vi "Pick&Place_ladder_shih_v7_center.vi"() -> ()   [LabVIEW 2016]
uses:
  WTF is this.ctl
  Classes/Controllers/I-O/Copy of NI-DAQ Folder/NI-DAQ.lvclass
  D:/INTT/V1/Classes/Controllers/I-O/Copy of I-O Folder/I-O.lvclass
  Classes/Controllers/Dispenser/Copy of Ultimus V2 Folder/Ultimus V2.lvclass
  <vilib>/Analysis/coordinate.llb/2D Cartesian Coordinate Rotation (Scalar).vi
  <vilib>/Utility/file.llb/Read Delimited Spreadsheet (DBL).vi
  <vilib>/Utility/file.llb/Write Delimited Spreadsheet (DBL).vi
  Classes/Controllers/Motion/Copy of Motion Folder/Motion.lvclass
  Classes/Controllers/Camera/Copy of Controller Folder/Controller.lvclass
  <vilib>/Analysis/NI_AALPro.lvlib
  Classes/Controllers/I-O/Copy of I-O Folder/I-O.lvclass
panel:
  in  "pick &place module":i32=1
  in  "txt switch":bool
  in  "offset":dbl[][](array[numeric])=[[0.0, 0.0, 0.0, 0.0], [0.0, 0.0, 0.0, 0.0]]
  out "HPoS_CT":dbl[][](array[numeric]) format="%#_8g"
  out "chip distance by OGP":dbl format="%#_8g"
  out "displacement":dbl[](array[numeric])
  out "gantry position test":dbl[](array[numeric])
  out "stave target position":dbl[](array[numeric])
  out "chip distance by gantry":dbl format="%#_8g"
  out "after SL":dbl[](array[numeric]) format="%#_8g"
  out "after SR":dbl[](array[numeric]) format="%#_8g"
  out "after NL":dbl[](array[numeric]) format="%#_8g"
  out "S chip":dbl[](array[numeric]) format="%#_8g"
  out "N chip":dbl[](array[numeric]) format="%#_8g"
  in  "file path (dialog if empty) 2":path=path "C:/Users/PAGANIS/Desktop/shih cheng wei/OGP/test1-2.txt"
  out "bless from OGP !!! Center of  stave":dbl[](array[numeric])
  out "bless from OGP !! measured stave size":dbl[](array[numeric])
  in  "Bless from OGP":bool
  out "FROM Detail !!! Center of module on stave":dbl[](array[numeric])
  out "FROM Detail !! measured stave size":dbl[](array[numeric])
  in  "Align Stave in detail":bool
  in  "check height?":bool
  in  "Uttimus presssure":i64=10
  out "Status":bool
  out "measured HDI top-left position":dbl[][](array[numeric])
  in  "HDI vacuum channel":i32=18
  in  "vacuum":bool=TRUE
  in  "HDI vacuum":bool
  out "measured stave size":dbl[](array[numeric])
  out "Stave mark":dbl[][](array[numeric])
  out "Center of module on stave":dbl[](array[numeric])
  out "Center of HDI from alignment mark":dbl[](array[numeric])
  out "Measured HDI size":dbl[][](array[numeric])
  out "module positions on stave":T1[][](array[typedef])
  in  "Default Stave dimension":dbl[](array[numeric])=[34.0, 472.0, -0.335295, -0.000320234]
  in  "Default Stave upper left mark":dbl[](array[numeric])=[584.376, 675.576, 70.9882, 0.000840064]
  out "Needle parking position":dbl[](array[numeric])
  in  "Uppler / Lower Stave":bool=TRUE
  out "Gantry current position":dbl[](array[numeric])
  in  "READ Position":bool
  in  "Needle Height Compenstation\n(glue gap)":dbl=0.33
  in  "Needle Alignment":bool
  in  "Parking position":dbl[](array[numeric])=[625.0, 625.0, 0.0, 0.01]
  in  "GOTO":bool
  in  "Default Pickup Tool Position":dbl[][](array[numeric])=[[152.226, 682.729, 36.8129, -0.0151898], [700.0, 800.0, 20.0, 0.01]]
  in  "deposit glue module":i32=1
  in  "Default HDI alignment \nmark position":dbl[](array[numeric])=[448.322, 976.582, 74.9872, 0.000191129]
  in  "Default HDI size":dbl[](array[numeric])=[24.2437, 231.446, -0.099339, 0.000191129]
  out "# of tasks excuted":i32
  out "HDI center positions":dbl[][](array[numeric])
  out "PickupTool \nCenterPosition":dbl[](array[numeric])
  in  "Inititalize":bool
  in  "Pick and place":bool
  in  "Deposit Glue":bool
  in  "Measure Pickup Tools":bool
  in  "Align Stave":bool
  out "default module position on stave":dbl[][](array[numeric])
  in  "Stop":bool
  in  "Measure HDI":bool
  # "Ladder Assembly"
  # "Lower\nmodule"
  # "Upper\nmodule"
  # "+"
  # "="
  # "Sensor 0.32 -> 200 micron glue thickness\nChips 0.37-> 140 micron glue thickness"
  # "ACTIONS"
  # "Stave infomation"
  # "also to switch Upper/Lower"
  # "theta had *-1"
  # "Module infomation"
  # "Pick and Place"
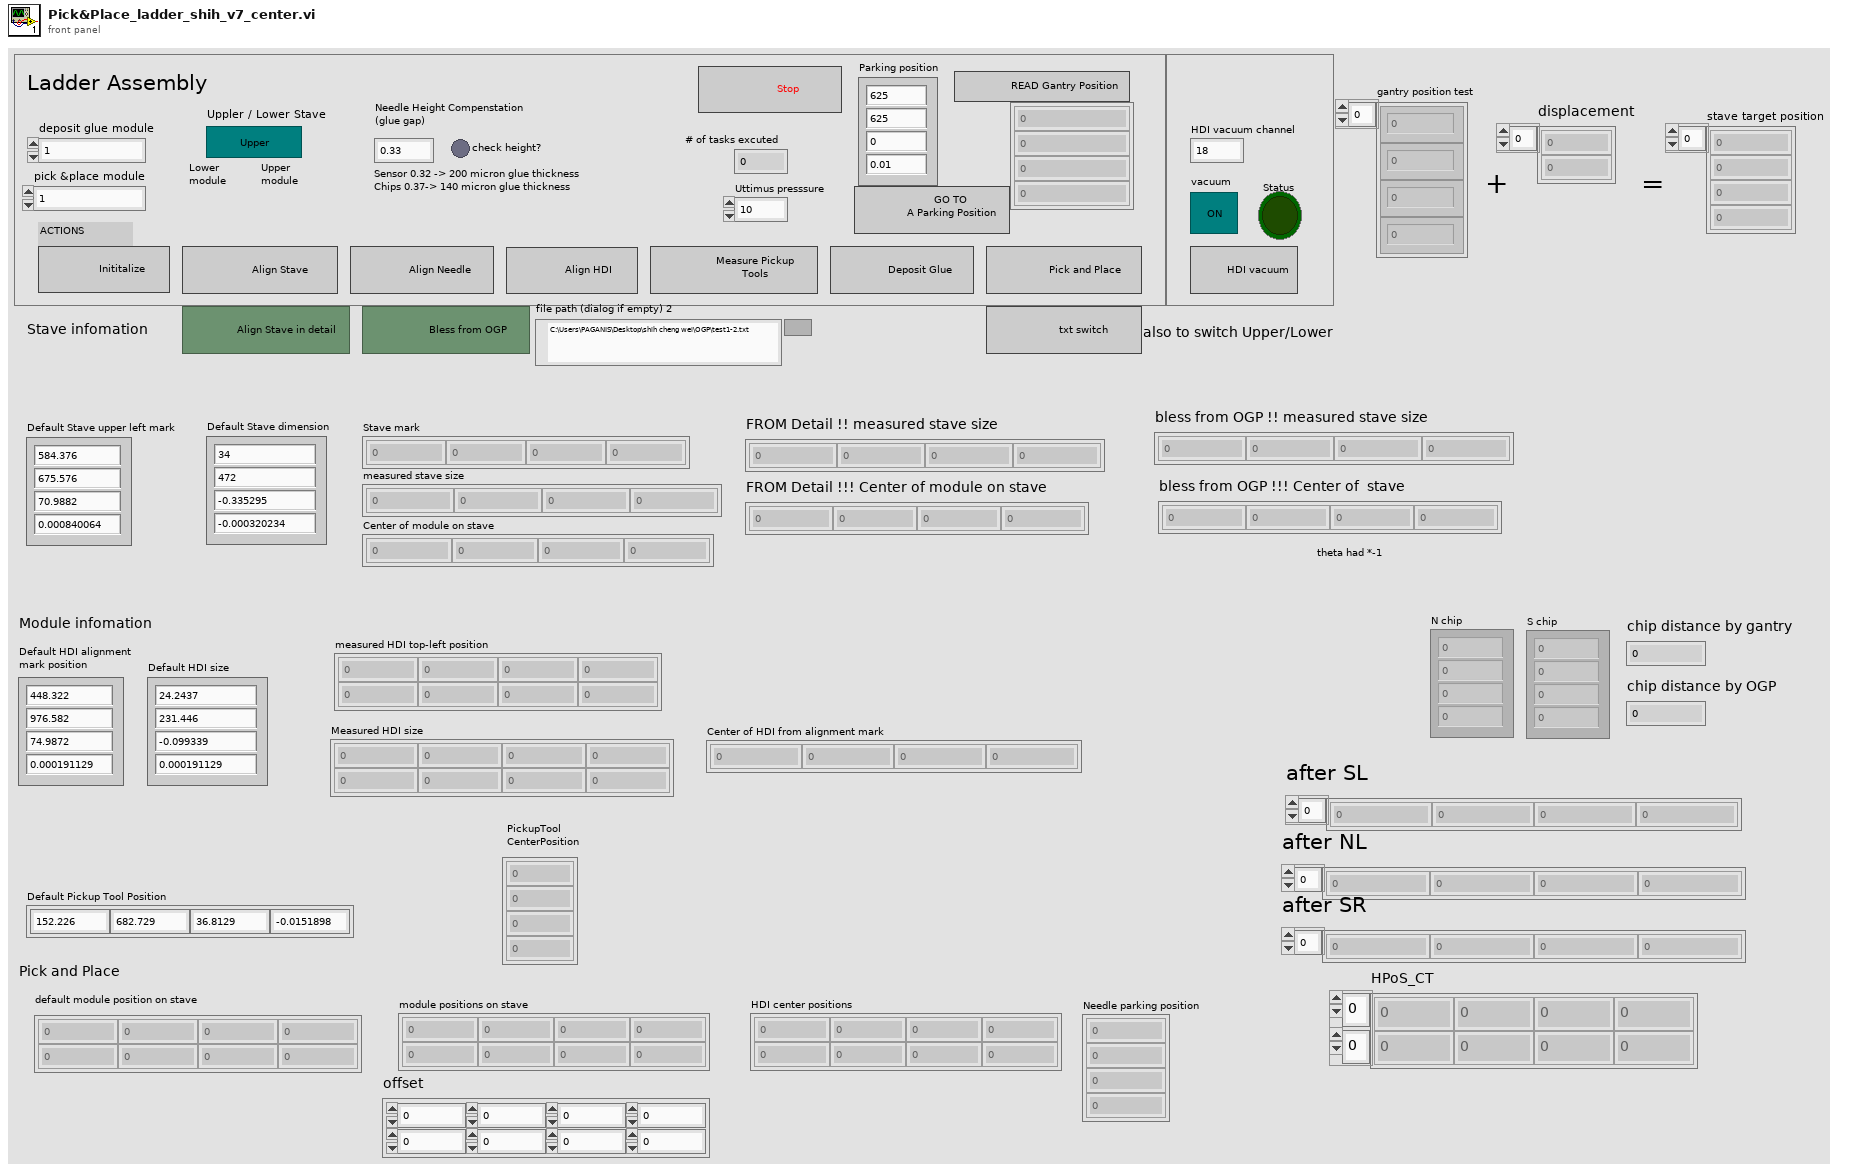
[diagram p1: front panel]
types:
  T1 = typedef "WTF is this.ctl" = dbl
  T2 = typedef "Controller.lvclass/Controllers.ctl" = cluster{"Copy of Motion.lvclass":refnum<class "Motion.lvclass">, "Copy of I-O.lvclass":refnum<class "I-O.lvclass">, "Copy of Dispenser.lvclass":refnum<class "Dispenser.lvclass">}
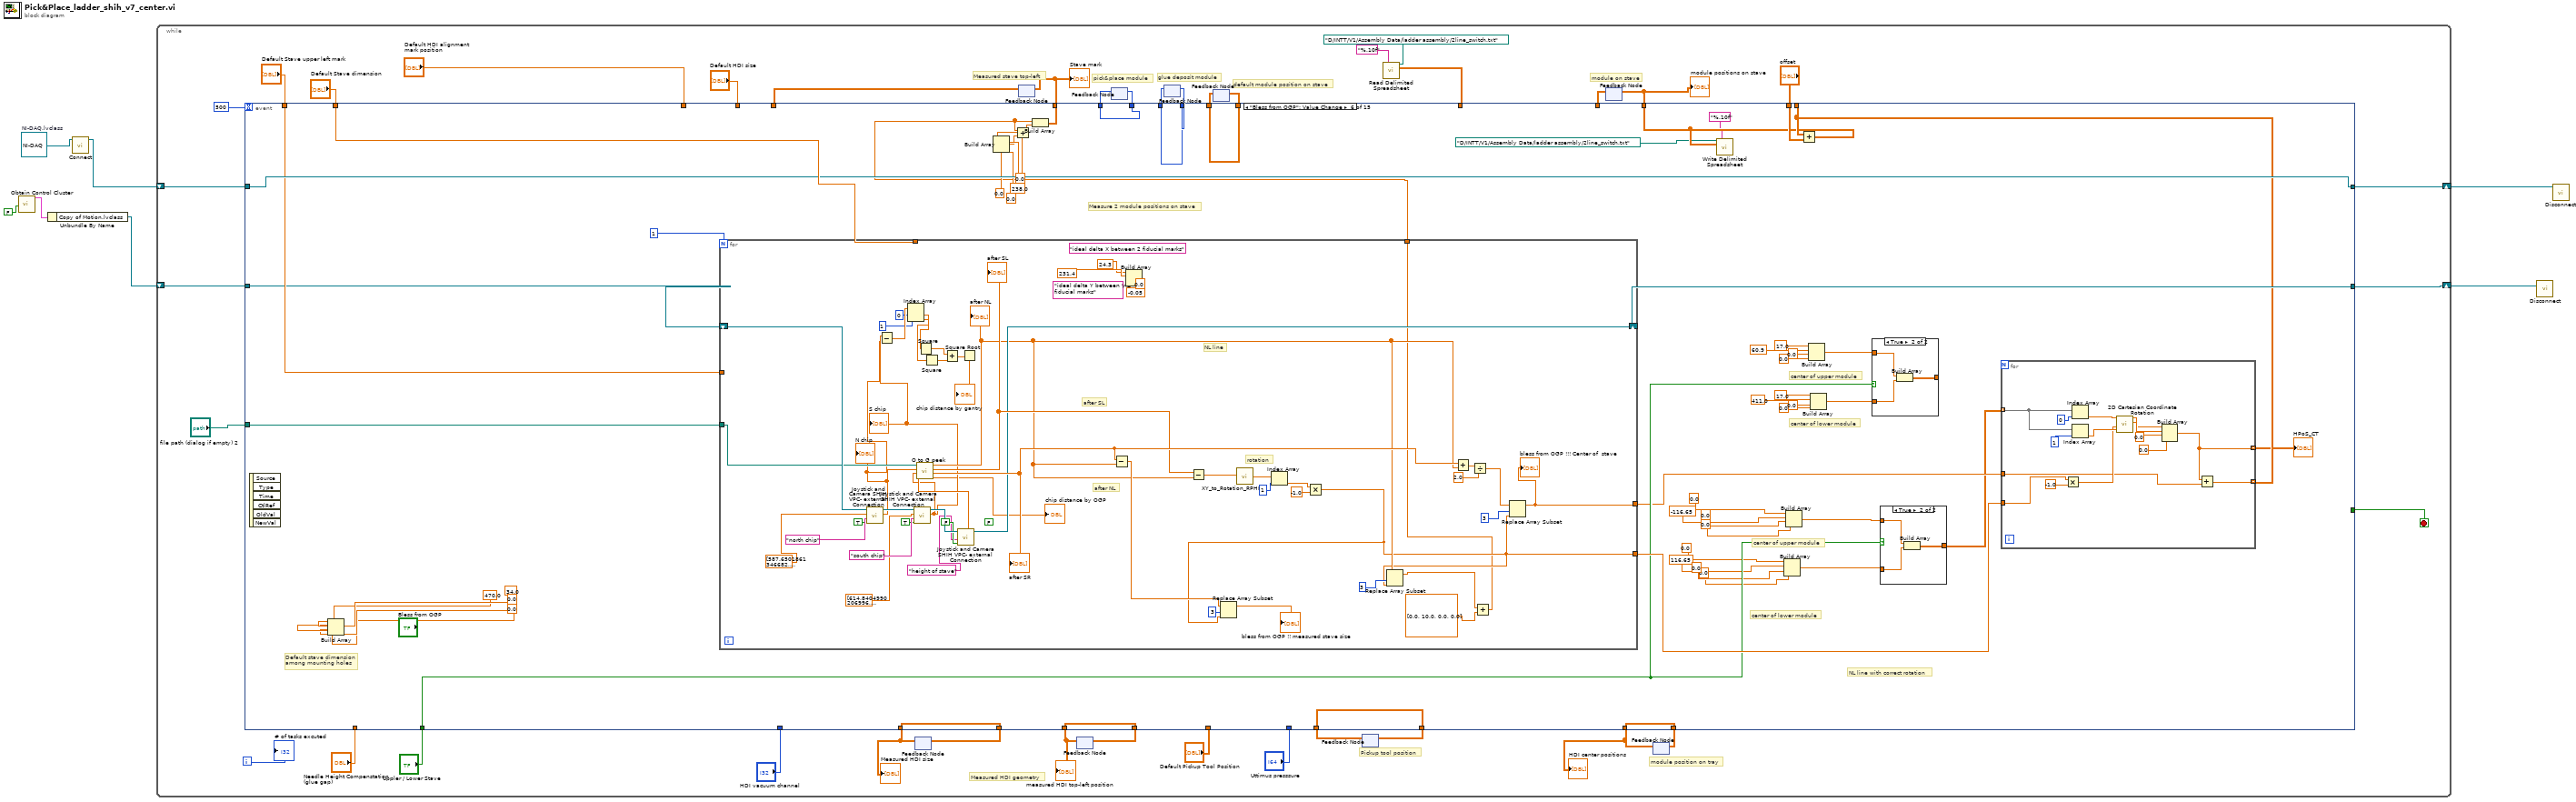
[diagram p0: block diagram]
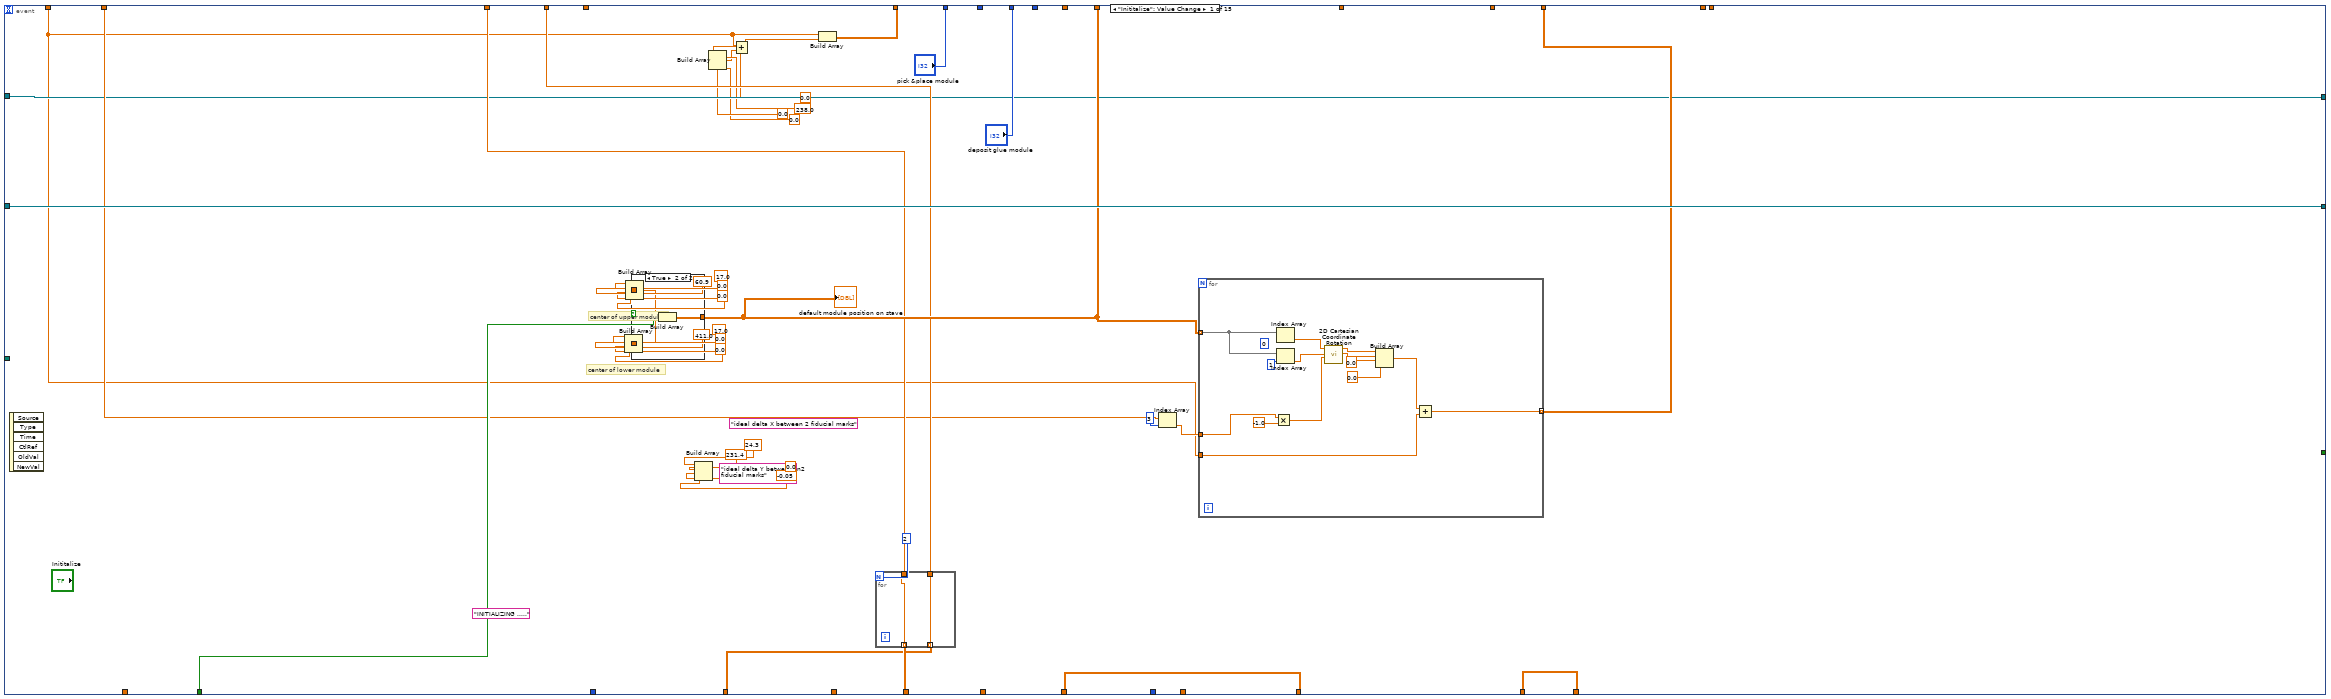
[diagram p2: hidden frame]
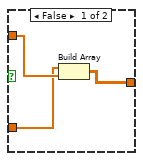
[diagram p3: hidden frame]
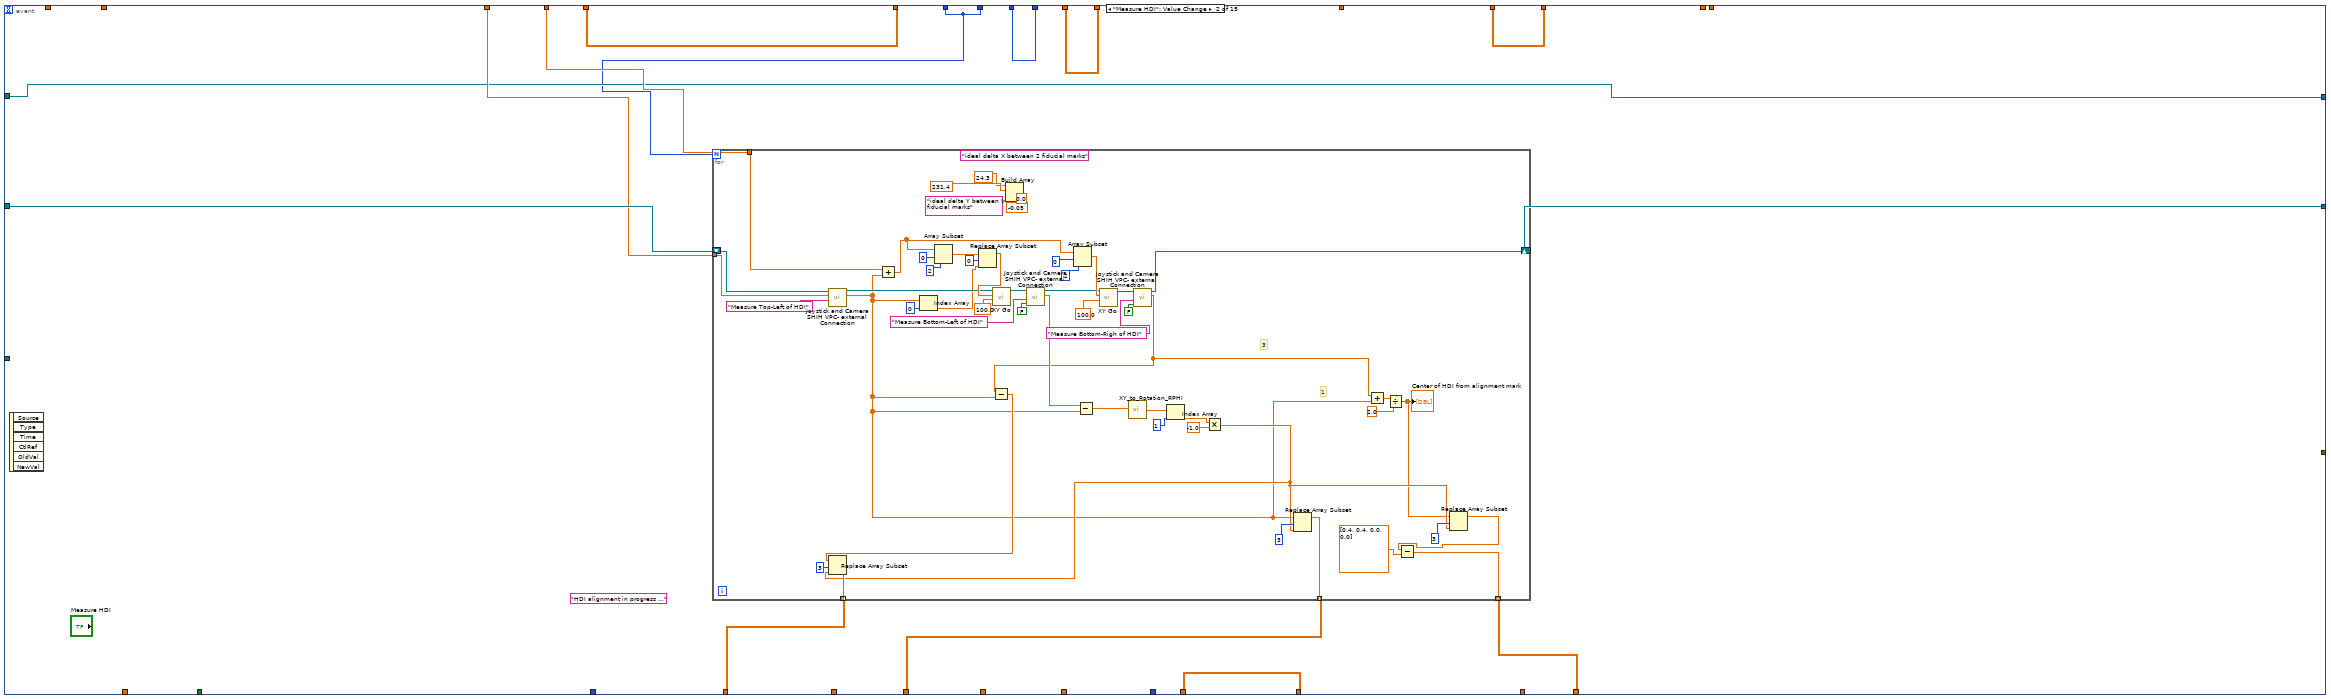
[diagram p4: hidden frame]
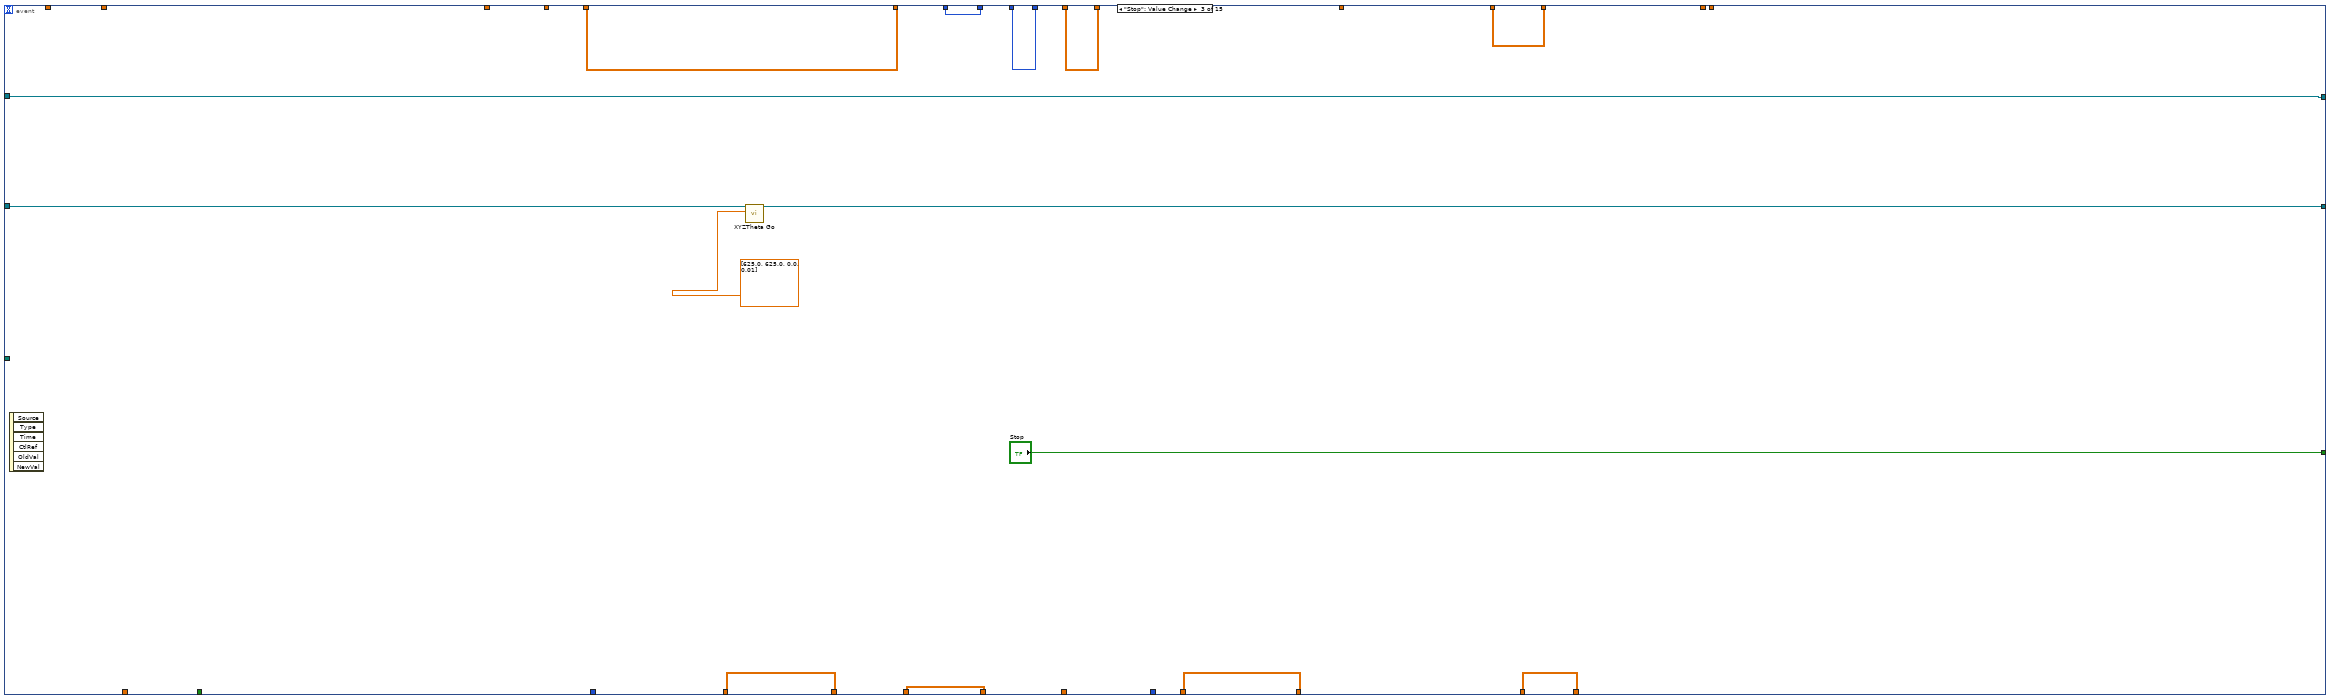
[diagram p5: hidden frame]
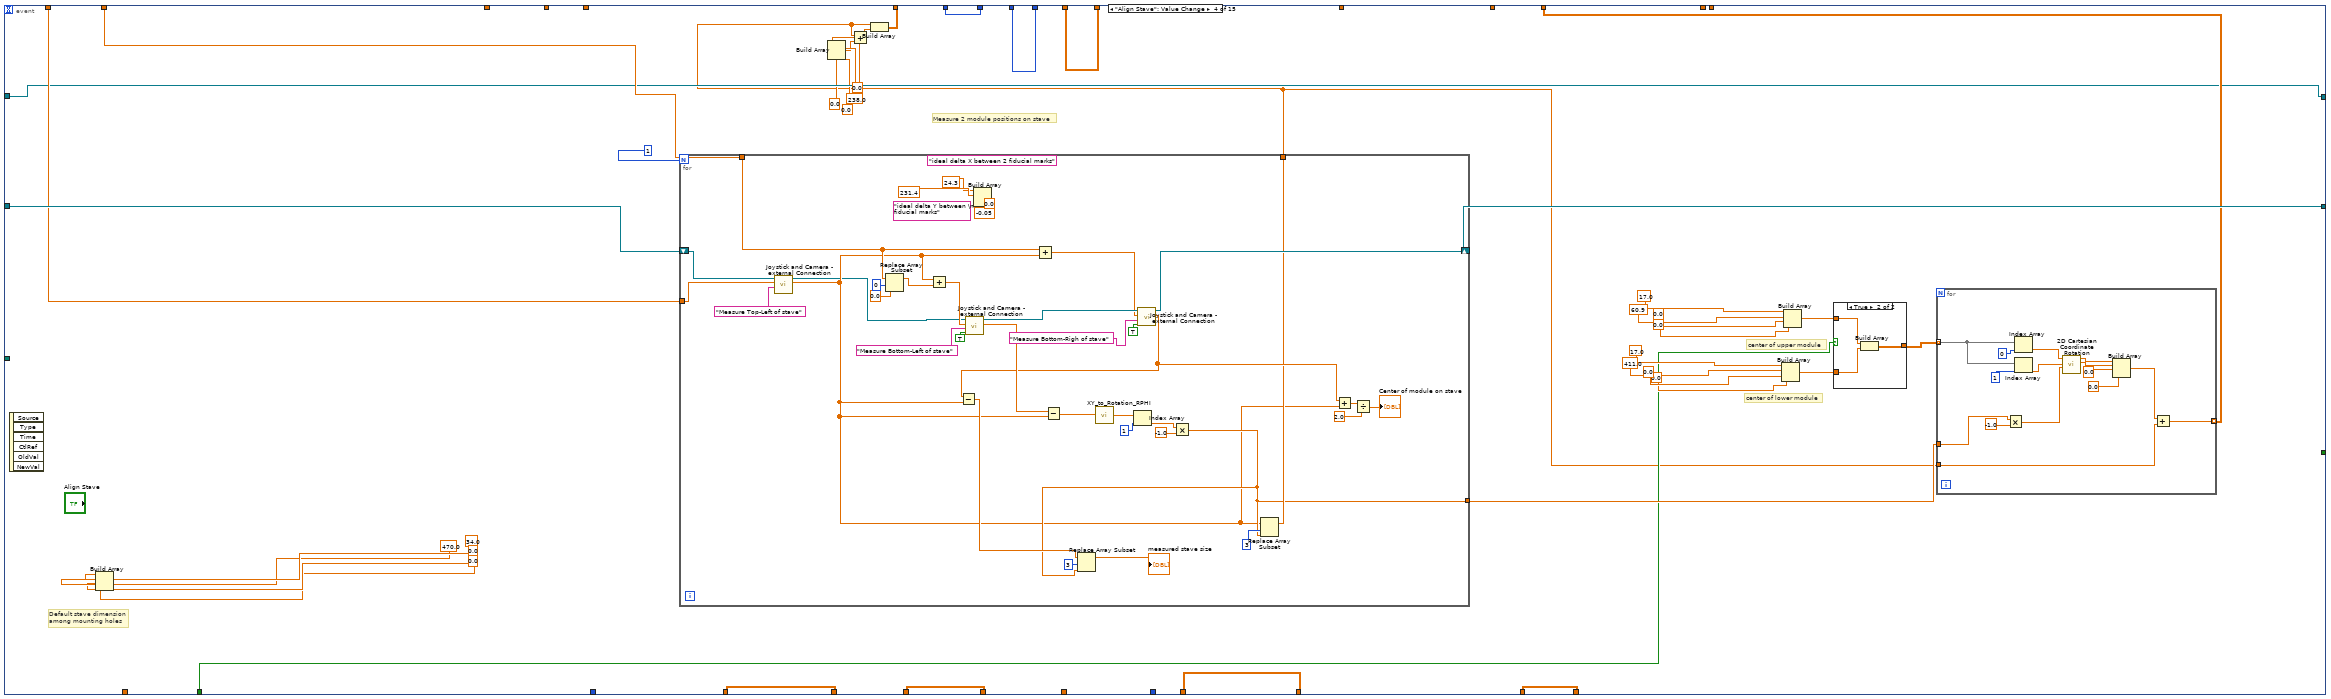
[diagram p6: hidden frame]
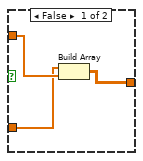
[diagram p7: hidden frame]
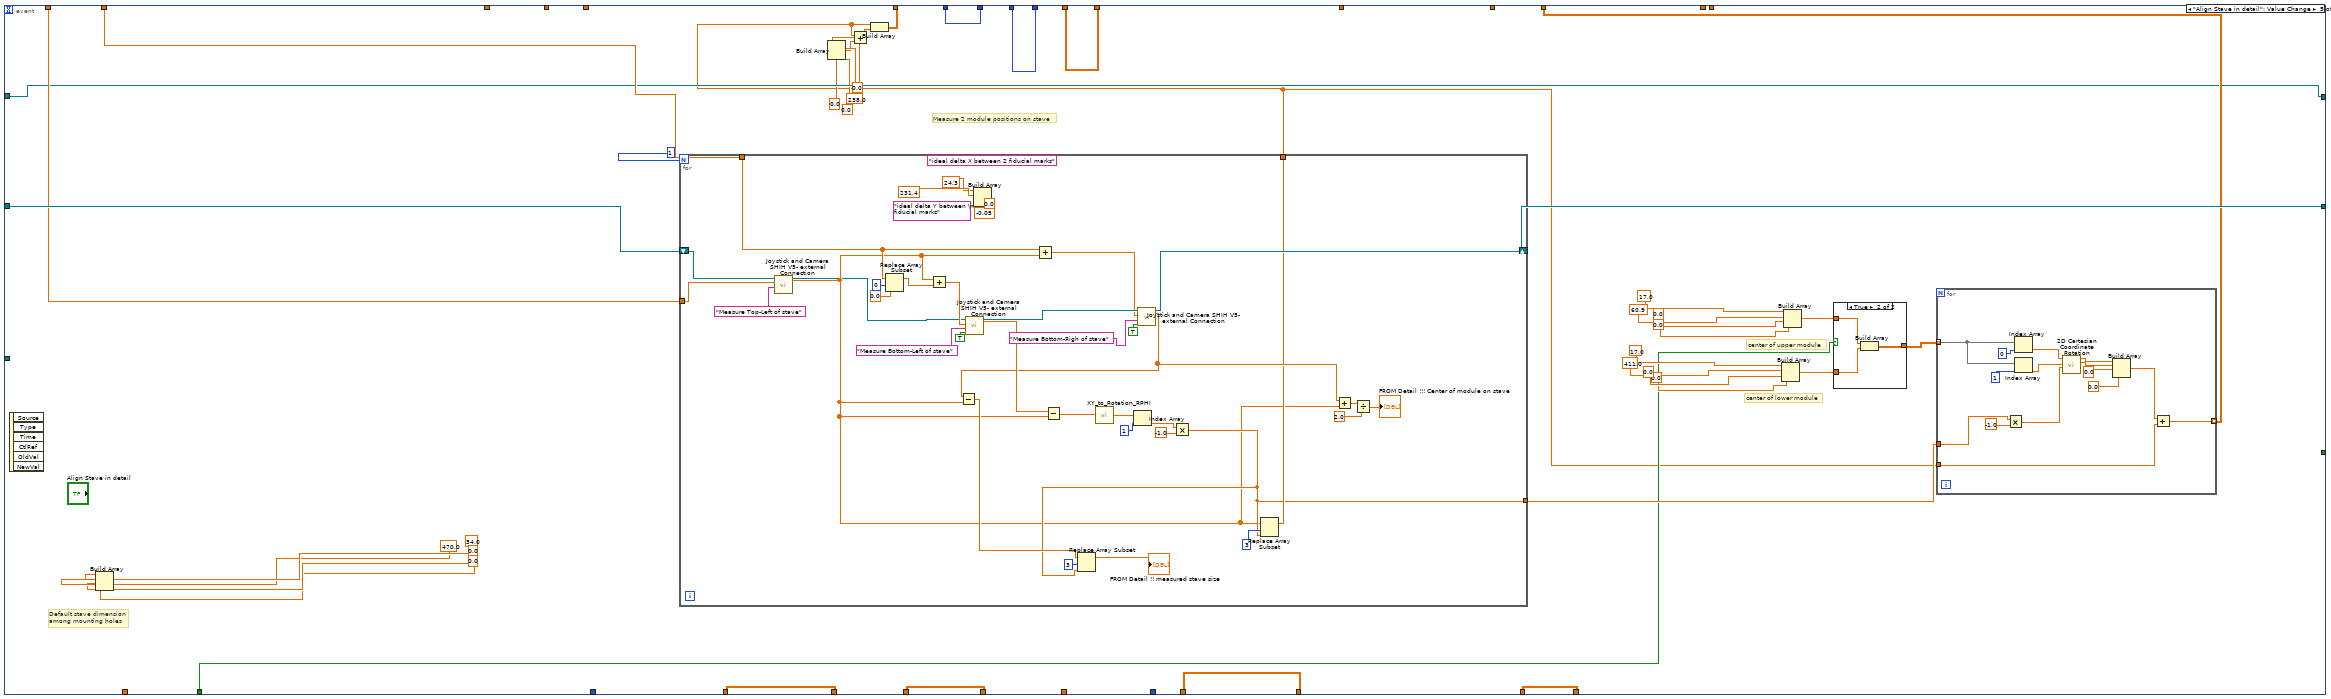
[diagram p8: hidden frame]
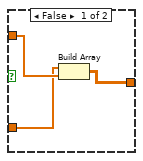
[diagram p9: hidden frame]
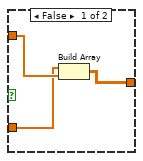
[diagram p10: hidden frame]
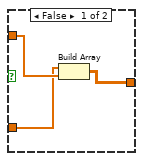
[diagram p11: hidden frame]
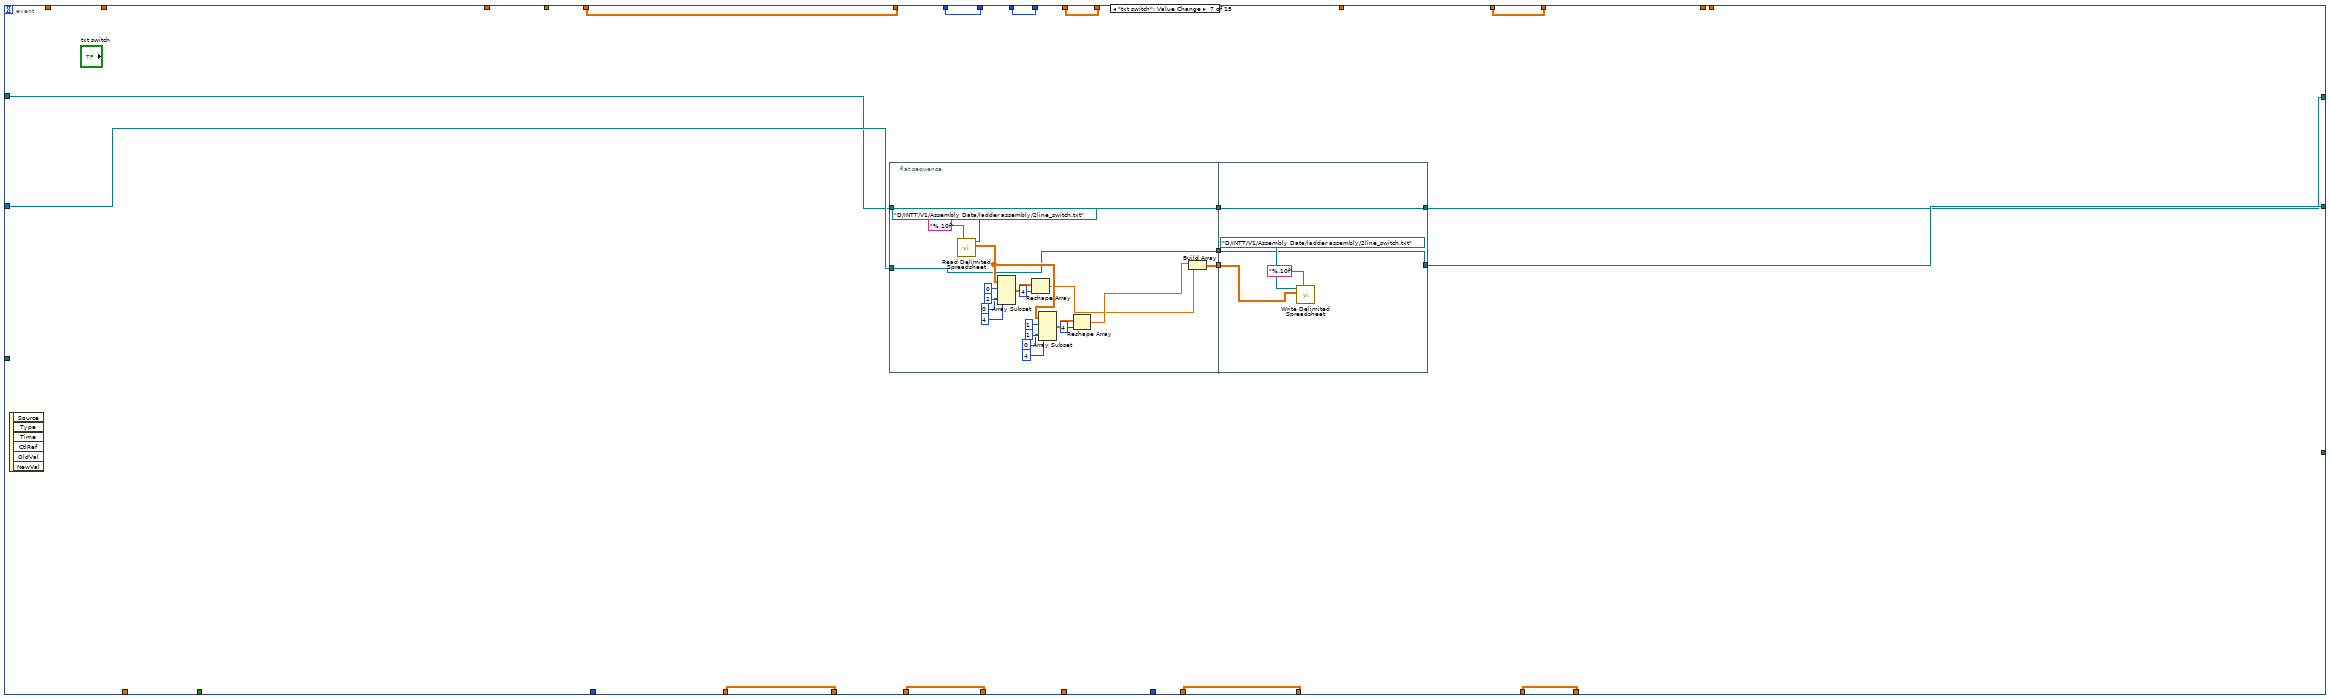
[diagram p12: hidden frame]
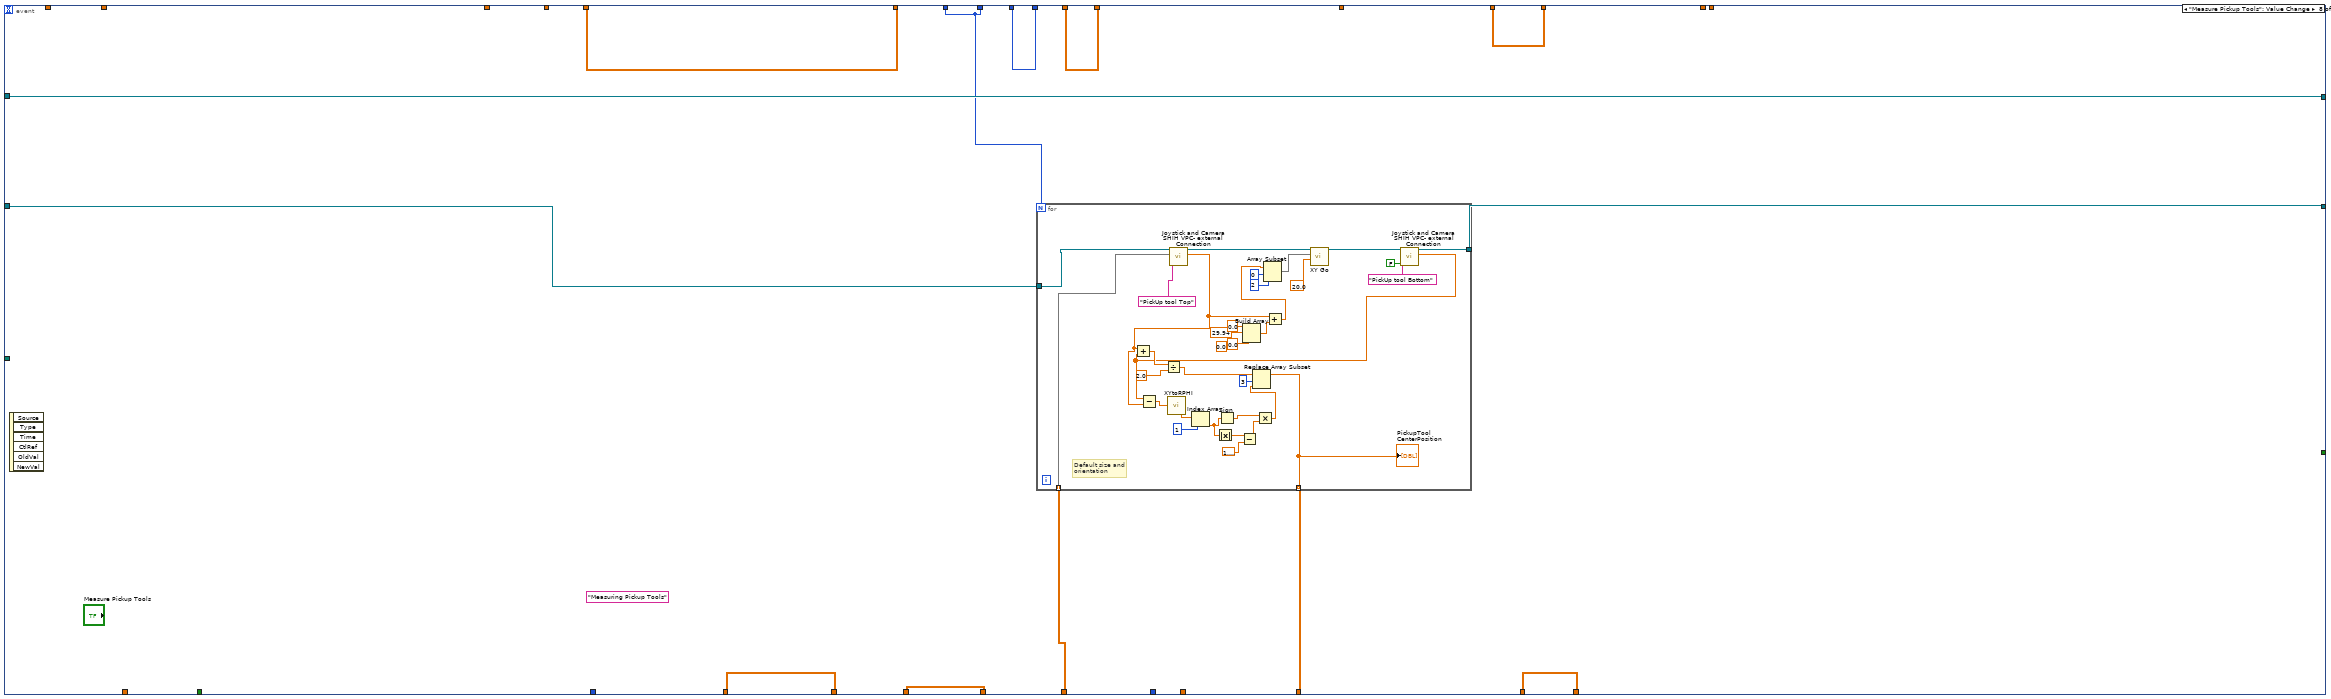
[diagram p13: hidden frame]
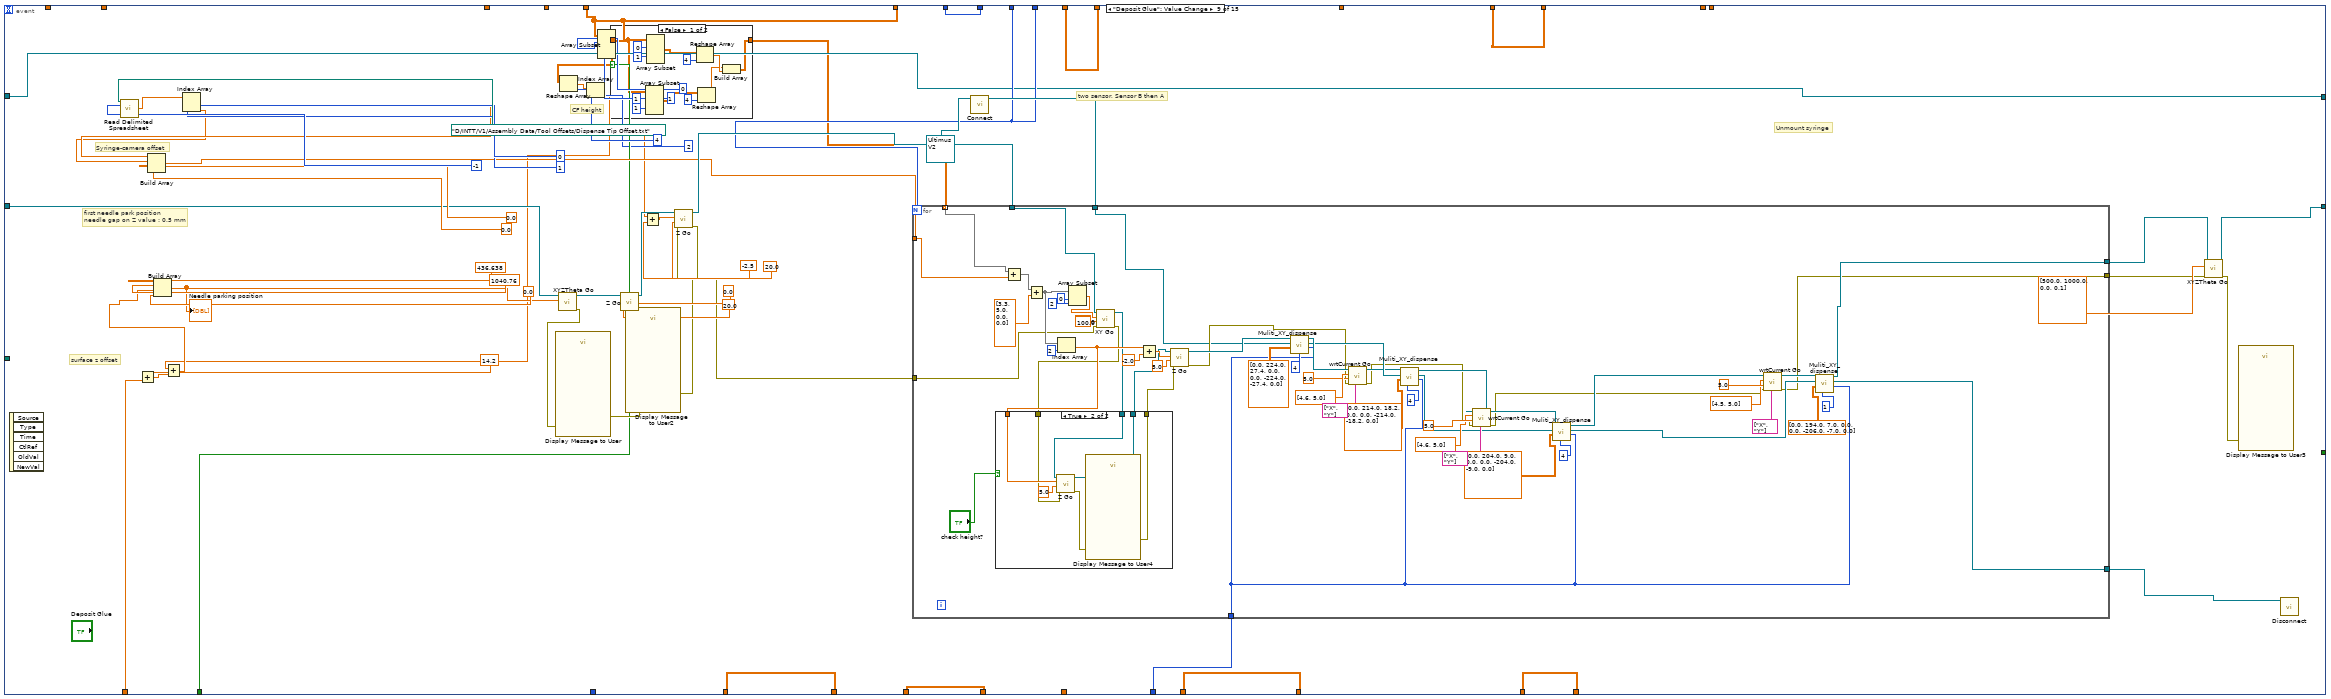
[diagram p14: hidden frame]
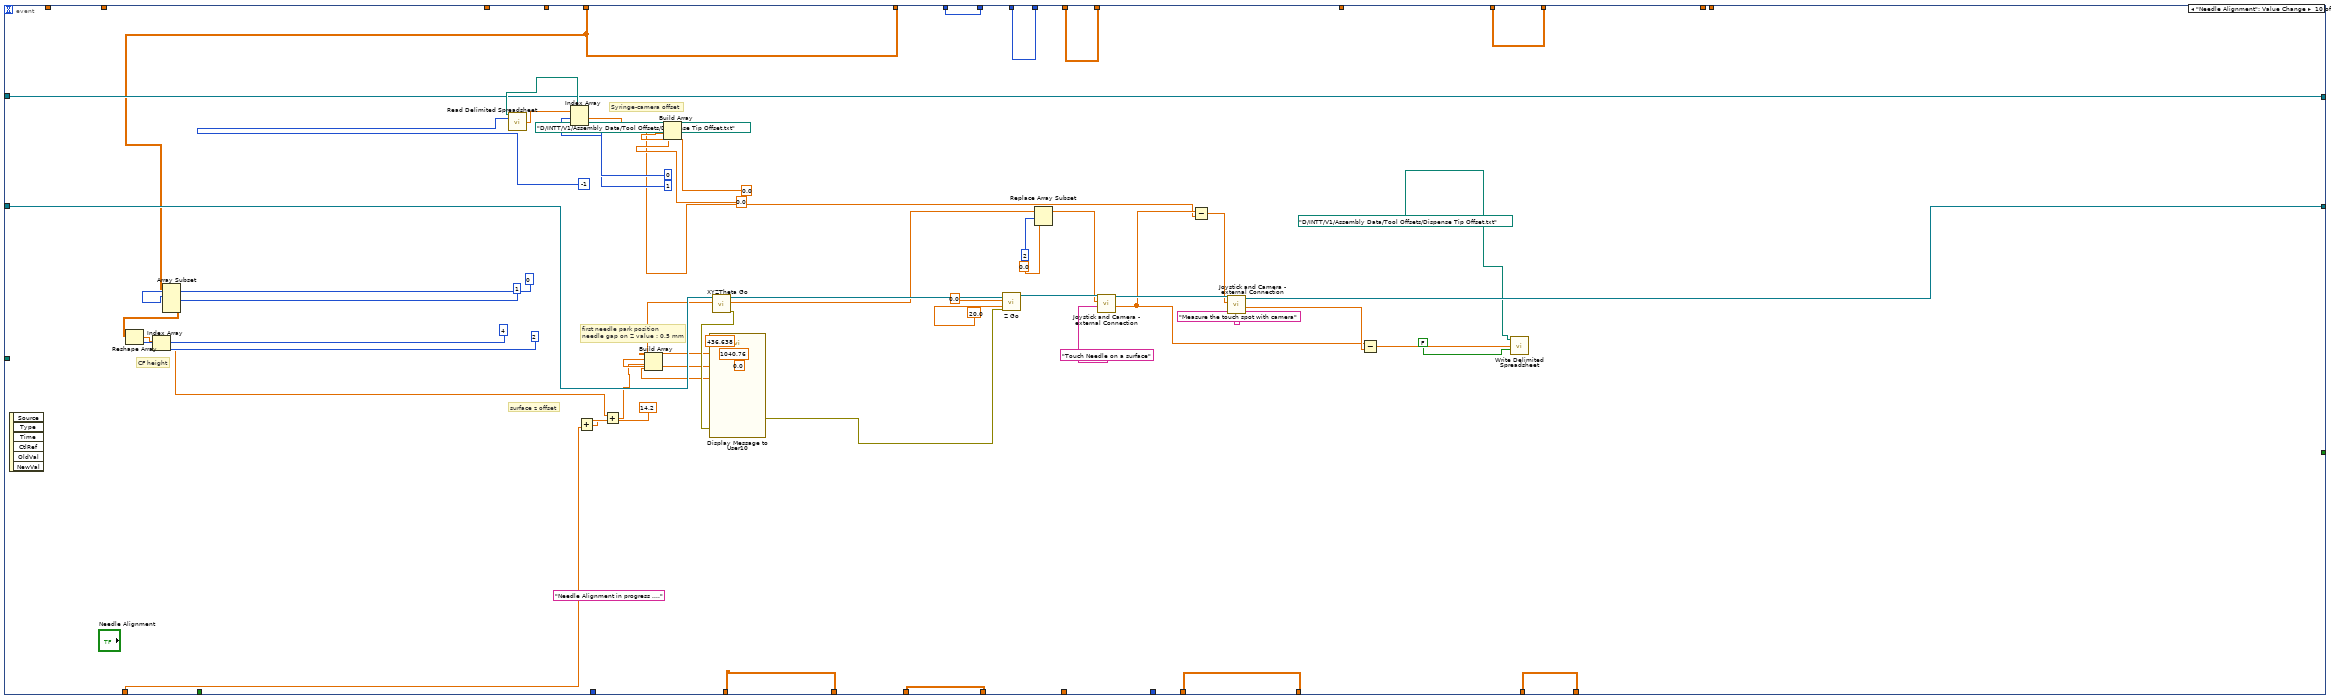
[diagram p17: hidden frame]
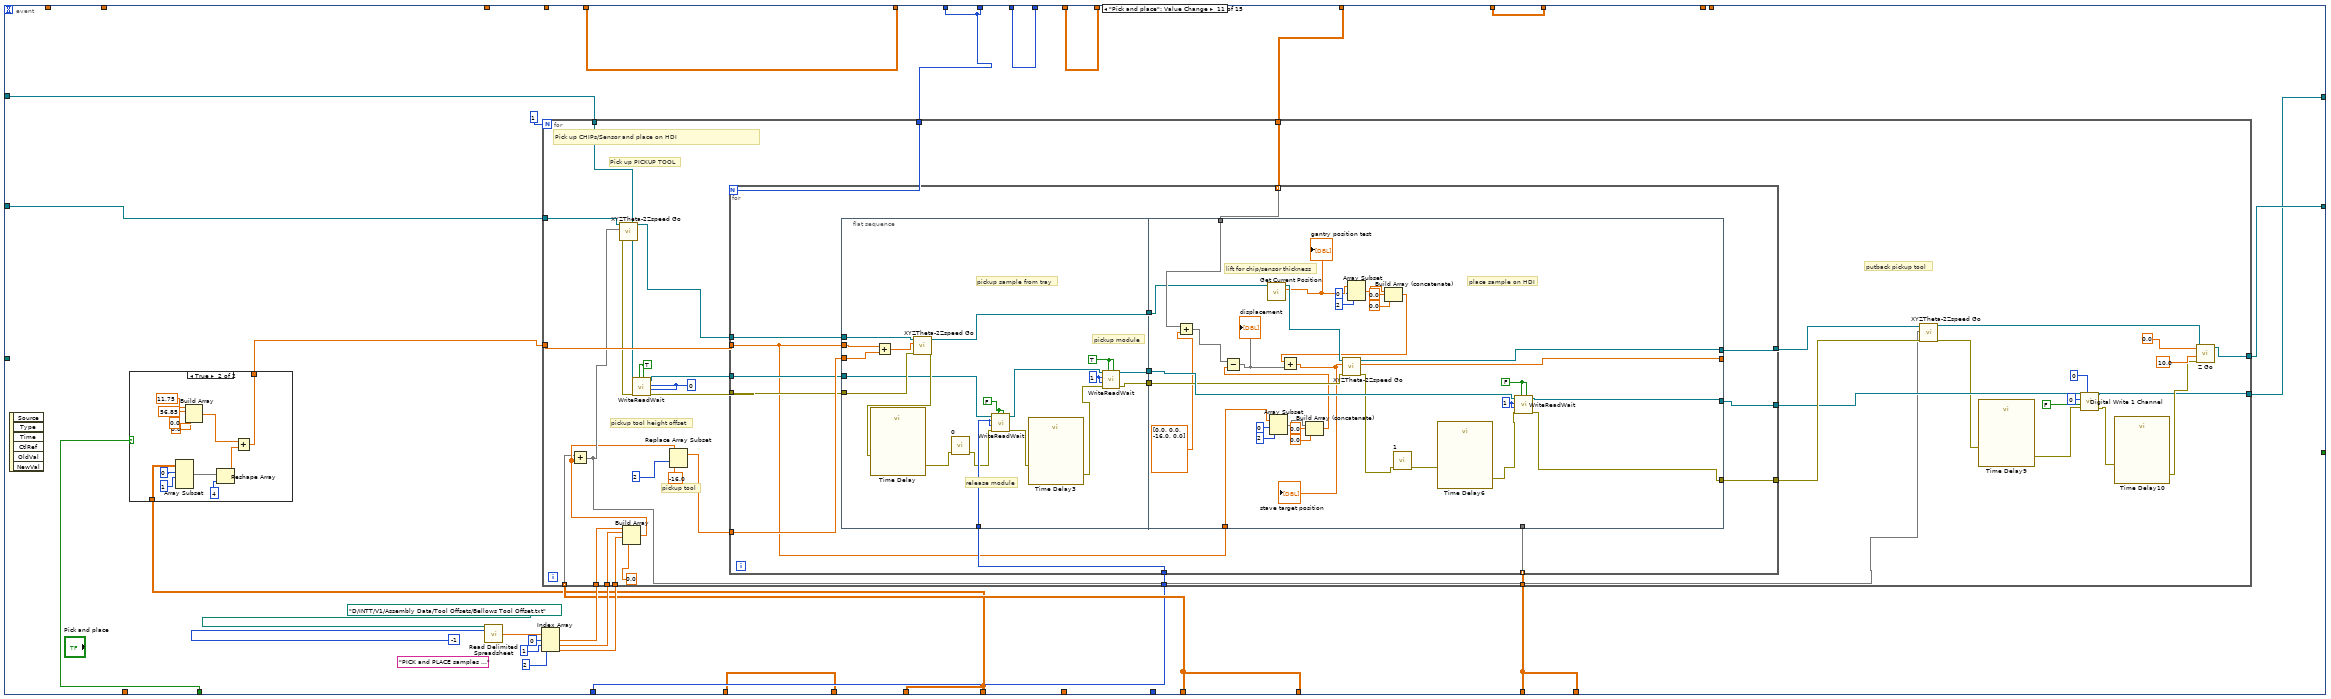
[diagram p18: hidden frame]
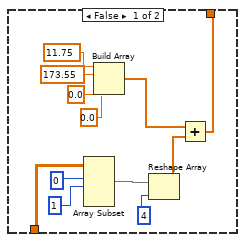
[diagram p19: hidden frame]
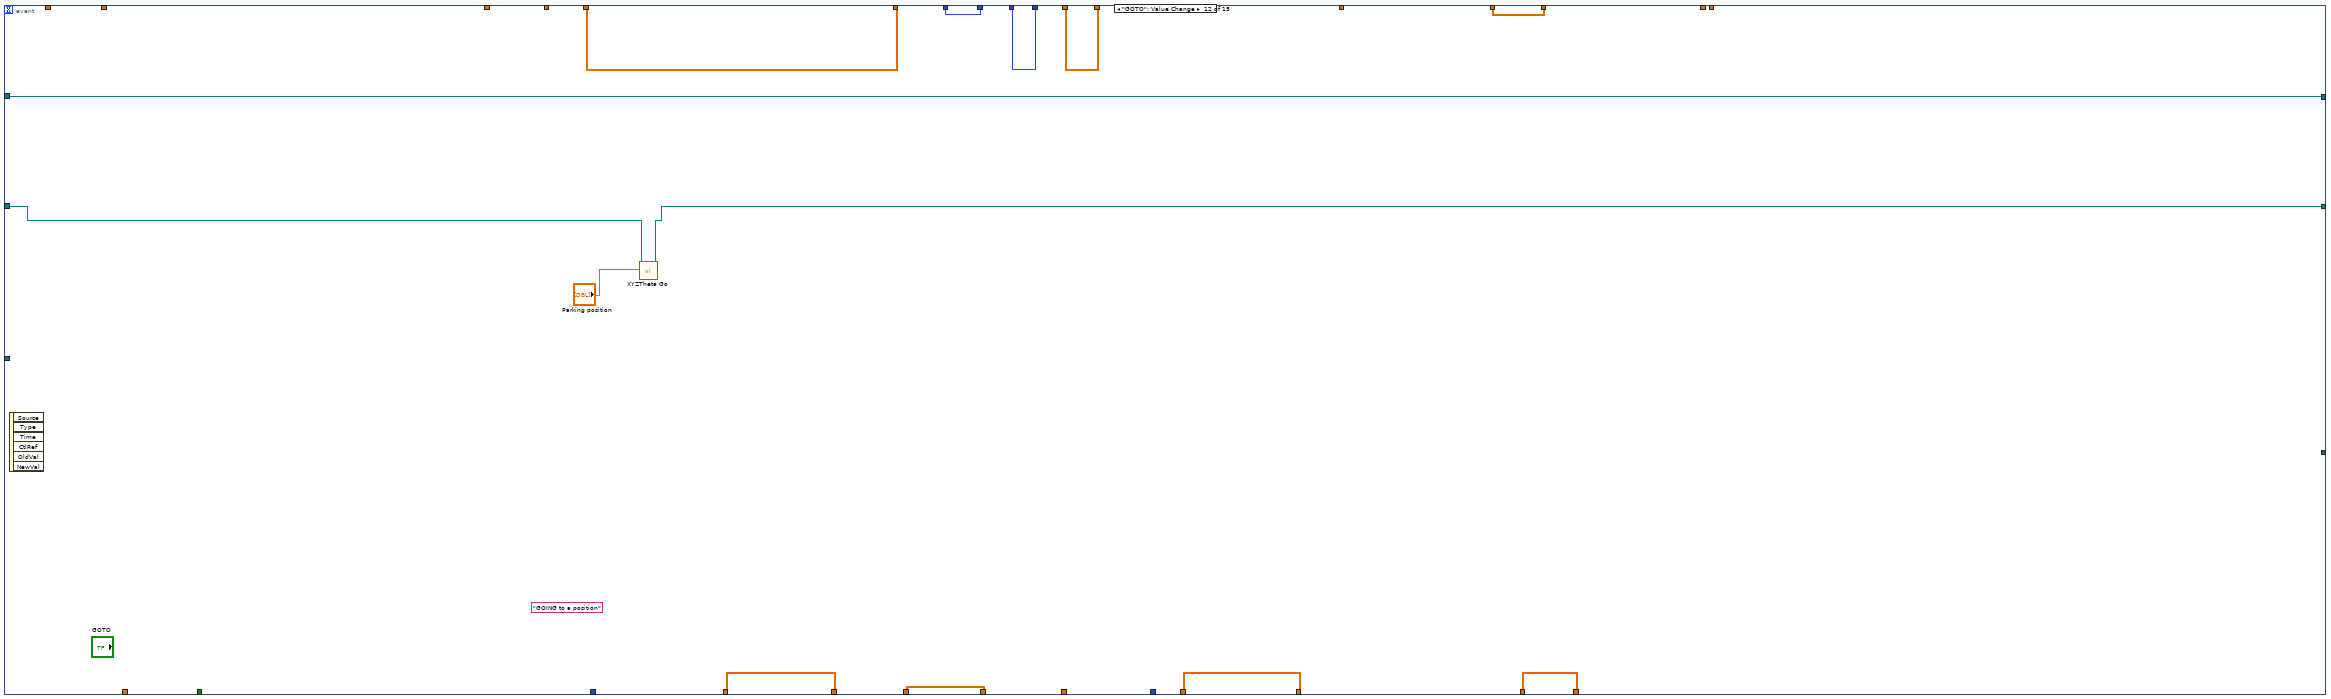
[diagram p20: hidden frame]
diagram:
  w3 = refnum<class "NI-DAQ.lvclass"> refnum  # NI-DAQ.lvclass
  n1 = call "Obtain Control Cluster.vi"("I/O"=FALSE) -> ("Control Out"=w7:T2)  [unwired: 10 in]
  n2 = Unbundle By Name(w7) -> ("Copy of Motion.lvclass"=w5:refnum<class "Motion.lvclass">)
  n3 = call-dynamic "Connect.vi"("NI-DAQ in"=w3) -> ("NI-DAQ out"=w2:refnum<class "NI-DAQ.lvclass">)  [unwired: 9 in, 1 out]
  n4 = while {
    shift-right: [w39] -> w4
    shift-left: w5 -> [w46]
    shift-right: [w18] -> w1
    shift-left: w2 -> [w22]
    i -> [w38]
    stop <- w45 stop-if-true
    # "pick&place module"
    # "default module position on stave"
    # "Pickup tool position"
    # "glue deposit module"
    # "Measured HDI geometry"
    # "module position on tray"
    # "Measured stave top-left"
    # "module on stave"
    n5 = feedback #1() -> (w43:dbl[][])  [unwired: 1 in]
    n6 = feedback #2() -> (w44:dbl[][])  [unwired: 1 in]
    n7 = feedback #3() -> (w19:dbl[][])  [unwired: 1 in]
    n8 = feedback #4() -> (w8:i32)  [unwired: 1 in]
    n9 = feedback #5() -> (w37:i32)  [unwired: 1 in]
    n10 = feedback #6() -> (w32:dbl[][])  [unwired: 1 in]
    n11 = feedback #7() -> (w40:dbl[][])  [unwired: 1 in]
    n12 = call-poly <vilib>:"Read Delimited Spreadsheet.vi"("file path (dialog if empty)"=path "D:/INTT/V1/Assembly Data/ladder assembly/2line_switch.txt" ("file path (dialog if empty) 3"), "format (%.3f)"="%.10f") -> ("all rows"=w10:dbl[][])  [unwired: 8 in, 5 out]
    n13 = feedback #8() -> (w26:dbl[][])  [unwired: 1 in]
    n14 = feedback #9() -> (w30:dbl[][])  [unwired: 1 in]
    "HDI center positions" <- w30
    n15 = event shown="[5] \"Bless from OGP\": Value Change" {
      selector: _ -> [_ _ _ _ _ _ _ _ _ _ _ _ _ _ _]
      dyn-events: _ -> [_ _ _ _ _ _ _ _ _ _ _ _ _ _ _]
      timeout: 500 -> [_ _ _ _ _ _ _ _ _ _ _ _ _ _ _]
      tunnel: w46 -> [w81 w121 w186 w217 w314 w411 w520 w568 w642 w777 w823 w957 w976 w979 w1001]
      tunnel: [_ _ "Stop" _ _ _ _ _ _ _ _ _ _ _ _] -> w45
      tunnel: [w48 w115 w181 w188 w285 w414 w525 w563 w604 w743 w804 w963 w972 w987 w1000] -> w23
      tunnel: w44 -> [_ w115 w181 _ _ _ w525 w563 w604 w743 w804 w963 w972 w987 w1000]
      tunnel: [w58 w113 w180 w213 w310 w426 w529 w562 w628 w780 w806 w960 w971 w981 w998] -> w24
      tunnel: w43 -> [_ _ w180 w213 w310 w426 w529 w562 w628 w780 w806 w960 w971 w981 w998]
      tunnel: w37 -> [_ w108 w183 w218 w315 w429 w524 w559 w631 w782 w800 w962 w973 w985 w992]
      tunnel: [w63 w112 w178 w220 w317 w431 w526 w561 w630 w778 w798 w958 w969 w983 w995] -> w42
      tunnel: w30 -> [w63 _ w178 w220 w317 w431 w526 w561 w630 w778 w798 w958 w969 w983 w995]
      tunnel: [w79 w116 w179 w225 w322 w436 w527 w567 w629 w779 w812 w959 w970 w982 w996] -> w41
      tunnel: w40 -> [_ w116 w179 w225 w322 w436 w527 _ w629 w779 w812 w959 w970 w982 w996]
      tunnel: [w81 w120 w184 w214 w311 w427 w518 w566 w632 w769 w813 w955 w975 w979 w1001] -> w39
      tunnel: ["deposit glue module" w108 w183 w218 w315 w429 w524 w559 w631 w782 w800 w962 w973 w985 w992] -> w36
      tunnel: "Default HDI alignment \nmark position" -> [w61 w119 _ _ _ _ _ _ _ _ _ _ _ _ _]
      tunnel: "Default HDI size" -> [w60 w118 _ _ _ _ _ _ _ _ _ _ _ _ _]
      tunnel: [w68 w117 w182 w219 w316 w430 w523 w564 w627 w781 w811 w961 w974 w986 w999] -> w33
      tunnel: w32 -> [_ w117 w182 w219 w316 w430 w523 w564 w627 w781 w811 w961 w974 w986 w999]
      tunnel: "Default Pickup Tool Position" -> [w79 _ _ _ _ _ _ w565 _ _ _ _ _ _ _]
      tunnel: "Uppler / Lower Stave" -> [w64 _ _ w198 w295 w409 _ _ w612 _ w799 _ _ _ _]
      tunnel: "Default Stave upper left mark" -> [w49 _ _ w216 w313 w413 _ _ _ _ _ _ _ _ _]
      tunnel: "Default Stave dimension" -> [w57 _ _ w215 w312 w428 _ _ _ _ _ _ _ _ _]
      tunnel: [w65 w114 w176 w197 w294 w394 w522 w560 w626 w760 w802 w953 w966 w984 w994] -> w25
      tunnel: w26 -> [_ w114 w176 _ _ _ w522 w560 w626 w760 w802 w953 w966 w984 w994]
      tunnel: w22 -> [w56 w110 w174 w196 w293 w422 w517 w557 w621 w758 w809 w952 w965 w991 w1004]
      tunnel: [w56 w110 w174 w196 w293 w422 w515 w557 w621 w758 w808 w952 w965 w978 w1002] -> w18
      tunnel: "HDI vacuum channel" -> [_ _ _ _ _ _ _ _ _ _ w807 _ _ w988 w1003]
      tunnel: [w59 w111 w175 w212 w309 w425 w528 w558 w622 w759 w805 w954 w967 w980 w997] -> w20
      tunnel: w19 -> [_ _ w175 w212 w309 w425 w528 w558 w622 w759 w805 w954 w967 w980 w997]
      tunnel: "Needle Height Compenstation\n(glue gap)" -> [_ _ _ _ _ _ _ _ w614 w751 _ _ _ _ _]
      tunnel: "Uttimus presssure" -> [_ _ _ _ _ _ _ _ w613 _ _ _ _ _ _]
      tunnel: "file path (dialog if empty) 2" -> [_ _ _ _ _ w412 _ _ _ _ _ _ _ _ _]
      tunnel: [_ _ _ _ _ w410 _ _ _ _ _ _ _ _ _] -> _
      tunnel: "offset" -> [_ _ _ _ _ w395 _ _ _ _ _ _ _ _ _]
      tunnel: w10 -> [_ _ _ _ _ _ _ _ _ _ w803 _ _ _ _]
      tunnel: ["pick &place module" w109 w173 w187 w284 w391 w521 w556 w603 w741 w801 w951 w964 w977 w993] -> w9
      tunnel: w8 -> [_ w109 w173 w187 w284 w391 w521 w556 w603 w741 w801 w951 w964 w977 w993]
      event "Inititalize": Value Change {
        (unwired) "INITIALIZING ....." ("String")
        (unwired) "ideal delta Y between \n2 fiducial marks"
        (unwired) "ideal delta X between 2 fiducial marks"
        # "center of lower module"
        # "center of upper module"
        n16 = event-data() -> ()  [unwired: 1 in, 6 out]
        n17 = Build Array(17.0 ("element"), 411.0 ("element"), 0.0 ("element"), 0.0 ("element")) -> (w69:dbl[])
        n18 = Build Array(17.0 ("element"), 60.9 ("element"), 0.0 ("element"), 0.0 ("element")) -> (w70:dbl[])
        n19 = case shown="True" w64 {
          tunnel: w70 -> [w90 w93]
          tunnel: w69 -> [w89 w92]
          tunnel: [w88 w91] -> w68
          frame False {
            n20 = Build Array(w89, w90) -> (w88:dbl[][])
          }
          frame True {
            n21 = Build Array(w93, w92) -> (w91:dbl[][])
          }
        }
        "default module position on stave" <- w68
        n22 = Build Array(24.3 ("y"), 231.4 ("y"), 0.0 ("element"), -0.05 ("element")) -> ()  [unwired: 1 out]
        n23 = Build Array(0.0 ("element"), 238.0 ("element"), 0.0 ("element"), 0.0 ("element")) -> (w51:dbl[])
        n24 = Add(x=w49, y=w51) -> (x+y=w50:dbl[])
        n25 = Build Array(w49, w50) -> (w48:dbl[][])
        n26 = for {
          N: 2 -> [_]
          tunnel: w61 -> [w87]
          tunnel: [w87] -> w59 mode=indexing
          tunnel: w60 -> [w86]
          tunnel: [w86] -> w58 mode=indexing
        }
        n27 = Index Array(array=w57, index=3) -> (element=w66:dbl)
        n28 = for {
          tunnel: w68 -> [w101] mode=indexing
          tunnel: w66 -> [w95]
          tunnel: w49 -> [w100]
          tunnel: [w98] -> w65 mode=indexing
          (unwired) 0 ("index")
          n29 = Multiply(x=w95, y=-1.0) -> (x*y=w96:dbl)
          n30 = Index Array(array=w101) -> (element=w104:dbl)  [unwired: 1 in]
          n31 = Index Array(array=w101, index=1) -> (element=w103:dbl)
          n32 = call-poly <vilib>:"2D Cartesian Coordinate Rotation.vi"("theta"=w96, "y"=w103, "x"=w104) -> ("y out"=w106:dbl, "x out"=w105:dbl)  [unwired: 6 in, 1 out]
          n33 = Build Array(w105, w106, 0.0 ("element"), 0.0 ("element")) -> (w99:dbl[])
          n34 = Add(x=w99, y=w100) -> (x+y=w98:dbl[])
        }
      }
      event "Measure HDI": Value Change {
        (unwired) "HDI alignment in progress ..." ("String")
        n35 = event-data() -> ()  [unwired: 1 in, 6 out]
        n36 = for {
          N: w109 -> [_]
          tunnel: w118 -> [w135]
          shift-right: [w132] -> w120
          shift-left: w121 -> [w133]
          tunnel: w119 -> [w134]
          tunnel: [w169] -> w111 mode=indexing
          tunnel: [w168] -> w113 mode=indexing
          tunnel: [w122] -> w112 mode=indexing
          (unwired) "ideal delta Y between \n2 fiducial marks"
          (unwired) "ideal delta X between 2 fiducial marks"
          # "1"
          # "3"
          n37 = call "Joystick and Camera SHIH VPC- external Connection.vi"("Motion in"=w133, "XYZTheta"=w134, "Measurement Point"="Measure Top-Left of HDI") -> ("Motion out"=w148:refnum<class "Motion.lvclass">, "Sum"=w125:dbl[])  [unwired: 4 in, 2 out]
          n38 = Add(x=w135, y=w125) -> (x+y=w152:dbl[])
          n39 = Index Array(array=w125, index=0) -> (element=w139:dbl)
          n40 = Array Subset(array=w152, index=0, length=2) -> (w151:dbl[])
          n41 = Replace Array Subset(array=w151, new element=w139, index=0) -> (w149:dbl[])
          n42 = call-dynamic "XY Go.vi"("Speed"=100.0, "XY"=w149, "Motion in"=w148) -> ("Motion out"=w156:refnum<class "Motion.lvclass">)  [unwired: 7 in, 1 out]
          n43 = Build Array(24.3 ("y"), 231.4 ("y"), 0.0 ("element"), -0.05 ("element")) -> ()  [unwired: 1 out]
          n44 = call "Joystick and Camera SHIH VPC- external Connection.vi"("Motion in"=w156, "Measurement Point"="Measure Bottom-Left of HDI", "Inital GO"=FALSE) -> ("Motion out"=w147:refnum<class "Motion.lvclass">, "Sum"=w138:dbl[])  [unwired: 4 in, 2 out]
          n45 = Array Subset(array=w152, index=0, length=2) -> (w162:dbl[])
          n46 = Subtract(x=w138, y=w125) -> (x-y=w146:dbl[])
          n47 = call-dynamic "XY Go.vi"("Speed"=100.0, "XY"=w162, "Motion in"=w147) -> ("Motion out"=w166:refnum<class "Motion.lvclass">)  [unwired: 7 in, 1 out]
          n48 = call "XY_to_Rotation_RPHI.vi"("X-Y"=w146) -> ("r-phi"=w142:dbl[])
          n49 = call "Joystick and Camera SHIH VPC- external Connection.vi"("Motion in"=w166, "Measurement Point"="Measure Bottom-Righ of HDI", "Inital GO"=FALSE) -> ("Motion out"=w132:refnum<class "Motion.lvclass">, "Sum"=w129:dbl[])  [unwired: 4 in, 2 out]
          n50 = Subtract(x=w129, y=w125) -> (x-y=w130:dbl[])
          n51 = Index Array(array=w142, index=1) -> (element=w136:dbl)
          n52 = Multiply(x=w136, y=-1.0) -> (x*y=w127:dbl)
          n53 = Replace Array Subset(array=w130, new element=w127, index=3) -> (w168:dbl[])
          n54 = Replace Array Subset(array=w125, new element=w127, index=3) -> (w169:dbl[])
          n55 = Add(x=w129, y=w125) -> (x+y=w171:dbl[])
          n56 = Divide(x=w171, y=2.0) -> (x/y=w126:dbl[])
          "Center of HDI from alignment mark" <- w126
          n57 = Replace Array Subset(array=w126, new element=w127, index=3) -> (w123:dbl[])
          n58 = Subtract(x=w123, y=dbl[] [0.4, 0.4, 0.0, 0.0]) -> (x-y=w122:dbl[])
        }
      }
      event "Stop": Value Change {
        n59 = event-data() -> ()  [unwired: 1 in, 6 out]
        n60 = call "XYZTheta Go.vi"("XYZTheta In"=dbl[] [625.0, 625.0, 0.0, 0.01], "Motion in"=w186) -> ("Motion out"=w184:refnum<class "Motion.lvclass">)  [unwired: 7 in, 2 out]
      }
      event "Align Stave": Value Change {
        # "center of lower module"
        # "center of upper module"
        # "Default stave dimension\namong mounting holes"
        # "Measure 2 module positions on stave"
        n61 = event-data() -> ()  [unwired: 1 in, 6 out]
        n62 = Build Array(34.0 ("element"), 470.0 ("element"), 0.0 ("element"), 0.0 ("element")) -> ()  [unwired: 1 out]
        n63 = for {
          N: 1 -> [_]
          tunnel: w215 -> [w232]
          shift-right: [w242] -> w214
          shift-left: w217 -> [w243]
          tunnel: w216 -> [w244]
          tunnel: [w237] -> w190
          tunnel: [w235] -> w200
          (unwired) "ideal delta Y between \n2 fiducial marks"
          (unwired) "ideal delta X between 2 fiducial marks"
          n64 = call "Joystick and Camera - external Connection.vi"("Motion in"=w243, "XYZTheta"=w244, "Measurement Point"="Measure Top-Left of stave") -> ("Motion out"=w226:refnum<class "Motion.lvclass">, "Sum"=w228:dbl[])  [unwired: 4 in, 2 out]
          n65 = Replace Array Subset(array=w232, new element=0.0 ("new element/subarray"), index=0) -> (w229:dbl[])
          n66 = Add(x=w228, y=w229) -> (x+y=w227:dbl[])
          n67 = call "Joystick and Camera - external Connection.vi"("Motion in"=w226, "XYZTheta"=w227, "Measurement Point"="Measure Bottom-Left of stave", "Inital GO"=TRUE) -> ("Motion out"=w234:refnum<class "Motion.lvclass">, "Sum"=w247:dbl[])  [unwired: 3 in, 2 out]
          n68 = Build Array(24.3 ("y"), 231.4 ("y"), 0.0 ("element"), -0.05 ("element")) -> ()  [unwired: 1 out]
          n69 = Add(x=w232, y=w228) -> (x+y=w233:dbl[])
          n70 = Subtract(x=w247, y=w228) -> (x-y=w253:dbl[])
          n71 = call "XY_to_Rotation_RPHI.vi"("X-Y"=w253) -> ("r-phi"=w249:dbl[])
          n72 = Index Array(array=w249, index=1) -> (element=w245:dbl)
          n73 = call "Joystick and Camera - external Connection.vi"("Motion in"=w234, "XYZTheta"=w233, "Measurement Point"="Measure Bottom-Righ of stave", "Inital GO"=TRUE) -> ("Motion out"=w242:refnum<class "Motion.lvclass">, "Sum"=w239:dbl[])  [unwired: 3 in, 2 out]
          n74 = Subtract(x=w239, y=w228) -> (x-y=w240:dbl[])
          n75 = Multiply(x=w245, y=-1.0) -> (x*y=w235:dbl)
          n76 = Replace Array Subset(array=w240, new element=w235, index=3) -> (→"measured stave size":dbl[])
          n77 = Replace Array Subset(array=w228, new element=w235, index=3) -> (w237:dbl[])
          n78 = Add(x=w239, y=w228) -> (x+y=w261:dbl[])
          n79 = Divide(x=w261, y=2.0) -> (x/y=→"Center of module on stave":dbl[])
        }
        n80 = Build Array(0.0 ("element"), 238.0 ("element"), 0.0 ("element"), 0.0 ("element")) -> (w191:dbl[])
        n81 = Add(x=w190, y=w191) -> (x+y=w189:dbl[])
        n82 = Build Array(w190, w189) -> (w188:dbl[][])
        n83 = Build Array(17.0 ("element"), 411.0 ("element"), 0.0 ("element"), 0.0 ("element")) -> (w202:dbl[])
        n84 = Build Array(17.0 ("element"), 60.9 ("element"), 0.0 ("element"), 0.0 ("element")) -> (w203:dbl[])
        n85 = case shown="True" w198 {
          tunnel: w203 -> [w280 w283]
          tunnel: w202 -> [w279 w282]
          tunnel: [w278 w281] -> w201
          frame False {
            n86 = Build Array(w279, w280) -> (w278:dbl[][])
          }
          frame True {
            n87 = Build Array(w283, w282) -> (w281:dbl[][])
          }
        }
        n88 = for {
          tunnel: w201 -> [w271] mode=indexing
          tunnel: w200 -> [w266]
          tunnel: w190 -> [w270]
          tunnel: [w268] -> w197 mode=indexing
          n89 = Multiply(x=w266, y=-1.0) -> (x*y=w265:dbl)
          n90 = Index Array(array=w271, index=0) -> (element=w274:dbl)
          n91 = Index Array(array=w271, index=1) -> (element=w273:dbl)
          n92 = call-poly <vilib>:"2D Cartesian Coordinate Rotation.vi"("theta"=w265, "y"=w273, "x"=w274) -> ("y out"=w276:dbl, "x out"=w275:dbl)  [unwired: 6 in, 1 out]
          n93 = Build Array(w275, w276, 0.0 ("element"), 0.0 ("element")) -> (w269:dbl[])
          n94 = Add(x=w269, y=w270) -> (x+y=w268:dbl[])
        }
      }
      event "Align Stave in detail": Value Change {
        # "center of lower module"
        # "center of upper module"
        # "Default stave dimension\namong mounting holes"
        # "Measure 2 module positions on stave"
        n95 = event-data() -> ()  [unwired: 1 in, 6 out]
        n96 = Build Array(34.0 ("element"), 470.0 ("element"), 0.0 ("element"), 0.0 ("element")) -> ()  [unwired: 1 out]
        n97 = for {
          N: 1 -> [_]
          tunnel: w312 -> [w329]
          shift-right: [w339] -> w311
          shift-left: w314 -> [w340]
          tunnel: w313 -> [w341]
          tunnel: [w334] -> w287
          tunnel: [w332] -> w297
          (unwired) "ideal delta Y between \n2 fiducial marks"
          (unwired) "ideal delta X between 2 fiducial marks"
          n98 = call "Joystick and Camera SHIH V5- external Connection.vi"("Motion in"=w340, "XYZTheta"=w341, "Measurement Point"="Measure Top-Left of stave") -> ("final out"=w325:dbl[], "Motion out"=w323:refnum<class "Motion.lvclass">)  [unwired: 5 in, 1 out]
          n99 = Replace Array Subset(array=w329, new element=0.0 ("new element/subarray"), index=0) -> (w326:dbl[])
          n100 = Add(x=w325, y=w326) -> (x+y=w324:dbl[])
          n101 = call "Joystick and Camera SHIH V5- external Connection.vi"("Motion in"=w323, "XYZTheta"=w324, "Measurement Point"="Measure Bottom-Left of stave", "Inital GO"=TRUE) -> ("final out"=w344:dbl[], "Motion out"=w331:refnum<class "Motion.lvclass">)  [unwired: 4 in, 1 out]
          n102 = Build Array(24.3 ("y"), 231.4 ("y"), 0.0 ("element"), -0.05 ("element")) -> ()  [unwired: 1 out]
          n103 = Add(x=w329, y=w325) -> (x+y=w330:dbl[])
          n104 = Subtract(x=w344, y=w325) -> (x-y=w350:dbl[])
          n105 = call "XY_to_Rotation_RPHI.vi"("X-Y"=w350) -> ("r-phi"=w346:dbl[])
          n106 = Index Array(array=w346, index=1) -> (element=w342:dbl)
          n107 = call "Joystick and Camera SHIH V5- external Connection.vi"("Motion in"=w331, "XYZTheta"=w330, "Measurement Point"="Measure Bottom-Righ of stave", "Inital GO"=TRUE) -> ("final out"=w336:dbl[], "Motion out"=w339:refnum<class "Motion.lvclass">)  [unwired: 4 in, 1 out]
          n108 = Subtract(x=w336, y=w325) -> (x-y=w337:dbl[])
          n109 = Multiply(x=w342, y=-1.0) -> (x*y=w332:dbl)
          n110 = Replace Array Subset(array=w337, new element=w332, index=3) -> (→"FROM Detail !! measured stave size":dbl[])
          n111 = Replace Array Subset(array=w325, new element=w332, index=3) -> (w334:dbl[])
          n112 = Add(x=w336, y=w325) -> (x+y=w358:dbl[])
          n113 = Divide(x=w358, y=2.0) -> (x/y=→"FROM Detail !!! Center of module on stave":dbl[])
        }
        n114 = Build Array(0.0 ("element"), 238.0 ("element"), 0.0 ("element"), 0.0 ("element")) -> (w288:dbl[])
        n115 = Add(x=w287, y=w288) -> (x+y=w286:dbl[])
        n116 = Build Array(w287, w286) -> (w285:dbl[][])
        n117 = Build Array(17.0 ("element"), 411.0 ("element"), 0.0 ("element"), 0.0 ("element")) -> (w299:dbl[])
        n118 = Build Array(17.0 ("element"), 60.9 ("element"), 0.0 ("element"), 0.0 ("element")) -> (w300:dbl[])
        n119 = case shown="True" w295 {
          tunnel: w300 -> [w377 w380]
          tunnel: w299 -> [w376 w379]
          tunnel: [w375 w378] -> w298
          frame False {
            n120 = Build Array(w376, w377) -> (w375:dbl[][])
          }
          frame True {
            n121 = Build Array(w380, w379) -> (w378:dbl[][])
          }
        }
        n122 = for {
          tunnel: w298 -> [w368] mode=indexing
          tunnel: w297 -> [w363]
          tunnel: w287 -> [w367]
          tunnel: [w365] -> w294 mode=indexing
          n123 = Multiply(x=w363, y=-1.0) -> (x*y=w362:dbl)
          n124 = Index Array(array=w368, index=0) -> (element=w371:dbl)
          n125 = Index Array(array=w368, index=1) -> (element=w370:dbl)
          n126 = call-poly <vilib>:"2D Cartesian Coordinate Rotation.vi"("theta"=w362, "y"=w370, "x"=w371) -> ("y out"=w373:dbl, "x out"=w372:dbl)  [unwired: 6 in, 1 out]
          n127 = Build Array(w372, w373, 0.0 ("element"), 0.0 ("element")) -> (w366:dbl[])
          n128 = Add(x=w366, y=w367) -> (x+y=w365:dbl[])
        }
      }
      event "Bless from OGP": Value Change {
        # "center of lower module"
        # "center of upper module"
        # "center of lower module"
        # "center of upper module"
        # "NL line with correct rotation"
        # "Default stave dimension\namong mounting holes"
        # "Measure 2 module positions on stave"
        n129 = event-data() -> ()  [unwired: 1 in, 6 out]
        n130 = Build Array(34.0 ("element"), 470.0 ("element"), 0.0 ("element"), 0.0 ("element")) -> ()  [unwired: 1 out]
        n131 = for {
          N: 1 -> [_]
          tunnel: w428 -> [_]
          shift-right: [w471] -> w427
          shift-left: w411 -> [w484]
          tunnel: w413 -> [_]
          tunnel: [w463] -> w416
          tunnel: [w466] -> w424
          tunnel: w412 -> [w473]
          tunnel: [w449] -> w398
          (unwired) FALSE ("Inital GO")
          (unwired) "ideal delta Y between \n2 fiducial marks"
          (unwired) "ideal delta X between 2 fiducial marks"
          # "after NL"
          # "after SL"
          # "NL line"
          # "rotation"
          n132 = call "Joystick and Camera SHIH VPC- external Connection.vi"("Motion in"=w484, "XYZTheta"=dbl[] [587.6501861346682, 659.8354057217969, 70.1155335060548, 0.010000094994154989] ("N chip"), "Measurement Point"="north chip", "Inital GO"=TRUE) -> ("Motion out"=w481:refnum<class "Motion.lvclass">, "Sum"=w461:dbl[])  [unwired: 3 in, 2 out]
          "N chip" <- w461
          n133 = call "Joystick and Camera SHIH VPC- external Connection.vi"("Motion in"=w481, "XYZTheta"=dbl[] [614.8404990206996, 1158.7590823829282, 70.34521582498871, 0.010000670236950445] ("S chip"), "Measurement Point"="south chip", "Inital GO"=TRUE) -> ("Motion out"=w480:refnum<class "Motion.lvclass">, "Sum"=w462:dbl[])  [unwired: 3 in, 2 out]
          "S chip" <- w462
          n134 = Subtract(x=w462, y=w461) -> (x-y=w460:dbl[])
          n135 = Index Array(array=w460, index #1=0 ("index"), index #2=1 ("index")) -> (element #1=w457:dbl, element #2=w456:dbl)
          n136 = Square(x=w457) -> (x^2=w454:dbl)
          n137 = Square(x=w456) -> (x^2=w455:dbl)
          n138 = Add(x=w454, y=w455) -> (x+y=w453:dbl)
          n139 = call "Joystick and Camera SHIH VPC- external Connection.vi"("Motion in"=w480, "Measurement Point"="height of stave", "Inital GO"=FALSE) -> ("Motion out"=w471:refnum<class "Motion.lvclass">, "Sum"=w472:dbl[])  [unwired: 4 in, 2 out]
          n140 = call "O to G peek.vi"("height"=w472, "south chip"=w462, "north chip"=w461, "Input file"=w473) -> ("OGP length"=→"chip distance by OGP":dbl, "output BR"=w475:dbl[], "output BL"=w474:dbl[], "output TL"=w468:dbl[])  [unwired: 4 in]
          "after NL" <- w468
          "after SR" <- w475
          "after SL" <- w474
          n141 = Square Root(x=w453) -> (sqrt(x)=→"chip distance by gantry":dbl)
          n142 = Subtract(x=w475, y=w468) -> (x-y=w486:dbl[])
          n143 = Build Array(24.3 ("y"), 231.4 ("y"), 0.0 ("element"), -0.05 ("element")) -> ()  [unwired: 1 out]
          n144 = Subtract(x=w474, y=w468) -> (x-y=w492:dbl[])
          n145 = call "XY_to_Rotation_RPHI.vi"("X-Y"=w492) -> ("r-phi"=w491:dbl[])
          n146 = Index Array(array=w491, index=1) -> (element=w488:dbl)
          n147 = Multiply(x=w488, y=-1.0) -> (x*y=w466:dbl)
          n148 = Replace Array Subset(array=w486, new element=w466, index=3) -> (→"bless from OGP !! measured stave size":dbl[])
          n149 = Replace Array Subset(array=w468, new element=w466, index=3) -> (w464:dbl[])
          n150 = Add(x=w475, y=w468) -> (x+y=w498:dbl[])
          n151 = Divide(x=w498, y=2.0) -> (x/y=w450:dbl[])
          n152 = Add(x=w464, y=dbl[] [0.0, 10.0, 0.0, 0.0]) -> (x+y=w463:dbl[])
          n153 = Replace Array Subset(array=w450, new element=w466, index=3) -> (w449:dbl[])
          "bless from OGP !!! Center of  stave" <- w449
        }
        n154 = Build Array(0.0 ("element"), 238.0 ("element"), 0.0 ("element"), 0.0 ("element")) -> (w417:dbl[])
        n155 = Add(x=w416, y=w417) -> (x+y=w415:dbl[])
        n156 = Build Array(w416, w415) -> (w414:dbl[][])
        n157 = Build Array(0.0 ("element"), 116.65 ("element"), 0.0 ("element"), 0.0 ("element")) -> (w399:dbl[])
        n158 = Build Array(0.0 ("element"), -116.65 ("element"), 0.0 ("element"), 0.0 ("element")) -> (w400:dbl[])
        n159 = Build Array(17.0 ("element"), 60.9 ("element"), 0.0 ("element"), 0.0 ("element")) -> (w382:dbl[])
        n160 = Build Array(17.0 ("element"), 411.0 ("element"), 0.0 ("element"), 0.0 ("element")) -> (w381:dbl[])
        n161 = case shown="True" w409 {
          tunnel: w382 -> [w439 w442]
          tunnel: w381 -> [w438 w441]
          tunnel: [w437 w440] -> _
          frame False {
            n162 = Build Array(w438, w439) -> (w437:dbl[][])
          }
          frame True {
            n163 = Build Array(w442, w441) -> (w440:dbl[][])
          }
        }
        n164 = case shown="True" w409 {
          tunnel: w400 -> [w445 w448]
          tunnel: w399 -> [w444 w447]
          tunnel: [w443 w446] -> w397
          frame False {
            n165 = Build Array(w444, w445) -> (w443:dbl[][])
          }
          frame True {
            n166 = Build Array(w448, w447) -> (w446:dbl[][])
          }
        }
        n167 = for {
          tunnel: w397 -> [w508] mode=indexing
          tunnel: w424 -> [w505]
          tunnel: [w507] -> w410 mode=indexing
          tunnel: w398 -> [w501]
          tunnel: [w500] -> w396 mode=indexing
          n168 = Multiply(x=w505, y=-1.0) -> (x*y=w504:dbl)
          n169 = Index Array(array=w508, index=0) -> (element=w511:dbl)
          n170 = Index Array(array=w508, index=1) -> (element=w510:dbl)
          n171 = call-poly <vilib>:"2D Cartesian Coordinate Rotation.vi"("theta"=w504, "y"=w510, "x"=w511) -> ("y out"=w513:dbl, "x out"=w512:dbl)  [unwired: 6 in, 1 out]
          n172 = Build Array(w512, w513, 0.0 ("element"), 0.0 ("element")) -> (w500:dbl[])
          n173 = Add(x=w500, y=w501) -> (x+y=w507:dbl[])
        }
        "HPoS_CT" <- w396
        n174 = Add(x=w410, y=w395) -> (x+y=w394:dbl[][])
        n175 = call-poly <vilib>:"Write Delimited Spreadsheet.vi"("file path (dialog if empty)"=path "D:/INTT/V1/Assembly Data/ladder assembly/2line_switch.txt", "format (%.3f)"="%.10f", "2D data"=w394) -> ()  [unwired: 11 in, 2 out]
      }
      event "txt switch": Value Change {
        n176 = event-data() -> ()  [unwired: 1 in, 6 out]
        n177 = flat-sequence {
          tunnel: [w536] -> w530
          tunnel: w520 -> [w532]
          tunnel: [w532] -> w519
          tunnel: w517 -> [w531]
          tunnel: [w531] -> w516
          tunnel: w530 -> [w554]
          tunnel: [w552] -> w518
          tunnel: w519 -> [w552]
          tunnel: [w551] -> w515
          tunnel: w516 -> [w551]
          frame #0 {
            n178 = call-poly <vilib>:"Read Delimited Spreadsheet.vi"("file path (dialog if empty)"=path "D:/INTT/V1/Assembly Data/ladder assembly/2line_switch.txt" ("file path (dialog if empty) 3"), "format (%.3f)"="%.10f") -> ("all rows"=w537:dbl[][])  [unwired: 8 in, 5 out]
            n179 = Array Subset(array=w537, index (row)=0 ("index"), length (row)=1 ("length"), index (col)=0 ("index"), length (col)=4 ("length")) -> (w547:dbl[][])
            n180 = Reshape Array(w547, 4 ("dimension size")) -> (w534:dbl[])
            n181 = Array Subset(array=w537, index (row)=1 ("index"), length (row)=1 ("length"), index (col)=0 ("index"), length (col)=4 ("length")) -> (w541:dbl[][])
            n182 = Reshape Array(w541, 4 ("dimension size")) -> (w535:dbl[])
            n183 = Build Array(w535, w534) -> (w536:dbl[][])
          }
          frame #1 {
            n184 = call-poly <vilib>:"Write Delimited Spreadsheet.vi"("file path (dialog if empty)"=path "D:/INTT/V1/Assembly Data/ladder assembly/2line_switch.txt" ("file path (dialog if empty) 4"), "format (%.3f)"="%.10f", "2D data"=w554) -> ()  [unwired: 11 in, 2 out]
          }
        }
      }
      event "Measure Pickup Tools": Value Change {
        (unwired) "Measuring Pickup Tools" ("String")
        n185 = event-data() -> ()  [unwired: 1 in, 6 out]
        n186 = for {
          N: w556 -> [_]
          tunnel: [w592] -> w567 mode=indexing
          tunnel: w568 -> [w596]
          tunnel: [w578] -> w566
          tunnel: w565 -> [w577] mode=indexing
          # "Default size and\norientation"
          n187 = call "Joystick and Camera SHIH VPC- external Connection.vi"("Motion in"=w596, "XYZTheta"=w577, "Measurement Point"="PickUp tool Top") -> ("Motion out"=w572:refnum<class "Motion.lvclass">, "Sum"=w595:dbl[])  [unwired: 4 in, 2 out]
          n188 = Build Array(0.0 ("element"), 29.94 ("element"), 0.0 ("element"), 0.0 ("element")) -> (w583:dbl[])
          n189 = Add(x=w595, y=w583) -> (x+y=w569:dbl[])
          n190 = Array Subset(array=w569, index=0, length=2) -> (w570:dbl[])
          n191 = call-dynamic "XY Go.vi"("Speed"=20.0, "XY"=w570, "Motion in"=w572) -> ("Motion out"=w571:refnum<class "Motion.lvclass">)  [unwired: 7 in, 1 out]
          n192 = call "Joystick and Camera SHIH VPC- external Connection.vi"("Motion in"=w571, "Measurement Point"="PickUp tool Bottom", "Inital GO"=FALSE) -> ("Motion out"=w578:refnum<class "Motion.lvclass">, "Sum"=w594:dbl[])  [unwired: 4 in, 2 out]
          n193 = Add(x=w595, y=w594) -> (x+y=w601:dbl[])
          n194 = Subtract(x=w594, y=w595) -> (x-y=w593:dbl[])
          n195 = Divide(x=w601, y=2.0) -> (x/y=w598:dbl[])
          n196 = call "XYtoRPHI.vi"("X-Y"=w593) -> ("r-phi"=w599:dbl[])
          n197 = Index Array(array=w599, index=1) -> (element=w587:dbl)
          n198 = Absolute Value(x=w587) -> (abs(x)=w590:dbl)
          n199 = Sign(1:w587) -> (0:w588:dbl)
          n200 = Subtract(x=w590, y=1.5707963267948966) -> (x-y=w589:dbl)
          n201 = Multiply(x=w588, y=w589) -> (x*y=w586:dbl)
          n202 = Replace Array Subset(array=w598, new element=w586, index=3) -> (w592:dbl[])
          "PickupTool \nCenterPosition" <- w592
        }
      }
      event "Deposit Glue": Value Change {
        # "CF height"
        # "surface z offset"
        # "two sensor, Sensor B then A"
        # "Unmount syringe"
        # "first needle park position\nneedle gap on Z value : 0.5 mm"
        # "Syringe-camera offset"
        n203 = event-data() -> ()  [unwired: 1 in, 6 out]
        n204 = call-poly <vilib>:"Read Delimited Spreadsheet.vi"("file path (dialog if empty)"=path "D:/INTT/V1/Assembly Data/Tool Offsets/Dispense Tip Offset.txt", "number of rows (all:-1)"=-1) -> ("first row"=w658:dbl[])  [unwired: 8 in, 5 out]
        n205 = Add(x=14.2 ("element"), y=w614) -> (x+y=w608:dbl)
        n206 = Index Array(array=w658, index #1=0 ("index"), index #2=1 ("index")) -> (element #1=w653:dbl, element #2=w651:dbl)
        n207 = Build Array(w653, w651, 0.0 ("element"), 0.0 ("element")) -> (w637:dbl[])
        n208 = Array Subset(array=w604, index (row)=0, length (row)=1 ("length")) -> (w617:dbl[][])  [unwired: 2 in]
        n209 = Reshape Array(w617, 4 ("dimension size")) -> (w610:dbl[])
        n210 = Index Array(array=w610, index=2) -> (element=w605:dbl)
        n211 = Add(x=w605, y=w608) -> (x+y=w607:dbl)
        n212 = Build Array(436.638, 1040.76, w607, 0.0 ("element")) -> (w606:dbl[])
        "Needle parking position" <- w606
        n213 = call "XYZTheta Go.vi"("XYZTheta In"=w606, "Motion in"=w642) -> ("error out"=w650:errorcluster, "Motion out"=w641:refnum<class "Motion.lvclass">)  [unwired: 7 in, 1 out]
        n214 = call "Display Message to User"("error in (no error)"=w650) -> ("error out"=w643:errorcluster)  [unwired: 9 in, 1 out]
        n215 = case shown="False" w612 {
          tunnel: w604 -> [w666 w675]
          tunnel: [w663 w675] -> w611
          frame False {
            n216 = Array Subset(array=w666, index (row)=1 ("index"), length (row)=1 ("length")) -> (w667:dbl[][])  [unwired: 2 in]
            n217 = Array Subset(array=w666, index (row)=0 ("index"), length (row)=1 ("length")) -> (w670:dbl[][])  [unwired: 2 in]
            n218 = Reshape Array(w670, 4 ("dimension size")) -> (w665:dbl[])
            n219 = Reshape Array(w667, 4 ("dimension size")) -> (w664:dbl[])
            n220 = Build Array(w664, w665) -> (w663:dbl[][])
          }
          frame True {
          }
        }
        n221 = call-dynamic "Z Go.vi"("error in (no error)"=w643, "Speed"=20.0, "Position"=0.0, "Motion in"=w641) -> ("error out"=w640:errorcluster, "Motion out"=w646:refnum<class "Motion.lvclass">)  [unwired: 6 in]
        n222 = call "Display Message to User2"("error in (no error)"=w640) -> ("error out"=w639:errorcluster)  [unwired: 9 in, 1 out]
        n223 = Add(x=w605, y=-2.5) -> (x+y=w647:dbl)
        n224 = call-dynamic "Z Go.vi"("error in (no error)"=w639, "Speed"=20.0, "Position"=w647, "Motion in"=w646) -> ("error out"=w616:errorcluster, "Motion out"=w638:refnum<class "Motion.lvclass">)  [unwired: 6 in]
        n225 = call-dynamic "Connect.vi"("Ultimus V in"=refnum<class "Ultimus V2.lvclass"> refnum ("Ultimus V2.lvclass")) -> ("Ultimus V out"=w636:refnum<class "Ultimus V2.lvclass">)  [unwired: 9 in, 1 out]
        n226 = for {
          N: w631 -> [_]
          tunnel: w638 -> [w690]
          tunnel: w636 -> [w689]
          tunnel: w637 -> [w691]
          tunnel: w611 -> [w692] mode=indexing
          tunnel: [w688] -> w624
          tunnel: [w687] -> w623
          tunnel: w616 -> [w683]
          tunnel: [w684] -> w615
          tunnel: w613 -> [w682]
          (unwired) 100.0 ("Speed")
          n227 = Add(x=w692, y=w691) -> (x+y=w722:dbl[])
          n228 = Add(x=w722, y=dbl[] [3.3, 5.0, 0.0, 0.0]) -> (x+y=w723:dbl[])
          n229 = Index Array(array=w723, index=2) -> (element=w680:dbl)
          n230 = Array Subset(array=w723, index=0, length=2) -> (w698:dbl[])
          n231 = call-dynamic "XY Go.vi"("error in (no error)"=w683, "Speed"=100.0, "XY"=w698, "Motion in"=w690) -> ("error out"=w678:errorcluster, "Motion out"=w679:refnum<class "Motion.lvclass">)  [unwired: 6 in]
          n232 = case shown="True" "check height?" {
            tunnel: w680 -> [_ w739]
            tunnel: w679 -> [w732 w738]
            tunnel: w678 -> [w733 w737]
            tunnel: [w733 w735] -> w677
            tunnel: [w732 w734] -> w676
            frame False {
            }
            frame True {
              n233 = call-dynamic "Z Go.vi"("error in (no error)"=w737, "Speed"=5.0, "Position"=w739, "Motion in"=w738) -> ("error out"=w736:errorcluster, "Motion out"=w734:refnum<class "Motion.lvclass">)  [unwired: 6 in]
              n234 = call "Display Message to User4"("error in (no error)"=w736) -> ("error out"=w735:errorcluster)  [unwired: 9 in, 1 out]
            }
          }
          n235 = Add(x=w680, y=-2.0) -> (x+y=w697:dbl)
          n236 = call-dynamic "Z Go.vi"("error in (no error)"=w677, "Speed"=5.0, "Position"=w697, "Motion in"=w676) -> ("error out"=w695:errorcluster, "Motion out"=w696:refnum<class "Motion.lvclass">)  [unwired: 6 in]
          n237 = call "Muliti_XY_dispense.vi"("Pressure"=w682, "Path count"=4, "distances"=dbl[][] [[0.0, 224.0], [27.4, 0.0], [0.0, -224.0], [-27.4, 0.0]], "Ultimus V in"=w689, "Motion in"=w696) -> ("Ultimus V out"=w716:refnum<class "Ultimus V2.lvclass">, "Motion out"=w721:refnum<class "Motion.lvclass">)  [unwired: 5 in]
          n238 = call-dynamic "wrtCurrent Go.vi"("axis names"=string[] ["X", "Y"], "error in (no error)"=w695, "Speed"=5.0, "distances"=dbl[] [4.6, 5.0], "Motion in"=w721) -> ("error out"=w686:errorcluster, "Motion out"=w715:refnum<class "Motion.lvclass">)  [unwired: 5 in]
          n239 = call "Muliti_XY_dispense.vi"("Pressure"=w682, "Path count"=4, "distances"=dbl[][] [[0.0, 214.0], [18.2, 0.0], [0.0, -214.0], [-18.2, 0.0]], "Ultimus V in"=w716, "Motion in"=w715) -> ("Ultimus V out"=w708:refnum<class "Ultimus V2.lvclass">, "Motion out"=w707:refnum<class "Motion.lvclass">)  [unwired: 5 in]
          n240 = call-dynamic "wrtCurrent Go.vi"("axis names"=string[] ["X", "Y"], "error in (no error)"=w686, "Speed"=5.0, "distances"=dbl[] [4.6, 5.0], "Motion in"=w707) -> ("error out"=w685:errorcluster, "Motion out"=w706:refnum<class "Motion.lvclass">)  [unwired: 5 in]
          n241 = call "Muliti_XY_dispense.vi"("Pressure"=w682, "Path count"=4, "distances"=dbl[][] [[0.0, 204.0], [9.0, 0.0], [0.0, -204.0], [-9.0, 0.0]], "Ultimus V in"=w708, "Motion in"=w706) -> ("Ultimus V out"=w693:refnum<class "Ultimus V2.lvclass">, "Motion out"=w694:refnum<class "Motion.lvclass">)  [unwired: 5 in]
          n242 = call-dynamic "wrtCurrent Go.vi"("axis names"=string[] ["X", "Y"], "error in (no error)"=w685, "Speed"=5.0, "distances"=dbl[] [4.5, 5.0], "Motion in"=w694) -> ("error out"=w684:errorcluster, "Motion out"=w700:refnum<class "Motion.lvclass">)  [unwired: 5 in]
          n243 = call "Muliti_XY_dispense.vi"("Pressure"=w682, "Path count"=1, "distances"=dbl[][] [[0.0, 194.0], [7.0, 0.0], [0.0, -206.0], [-7.0, 0.0]], "Ultimus V in"=w693, "Motion in"=w700) -> ("Ultimus V out"=w687:refnum<class "Ultimus V2.lvclass">, "Motion out"=w688:refnum<class "Motion.lvclass">)  [unwired: 5 in]
        }
        n244 = call "XYZTheta Go.vi"("error in (no error)"=w615, "XYZTheta In"=dbl[] [500.0, 1000.0, 0.0, 0.1], "Motion in"=w624) -> ("error out"=w634:errorcluster, "Motion out"=w632:refnum<class "Motion.lvclass">)  [unwired: 6 in, 1 out]
        n245 = call "Display Message to User3"("error in (no error)"=w634) -> ()  [unwired: 9 in, 2 out]
        n246 = call-dynamic "Disconnect.vi"("Ultimus V in"=w623) -> ()  [unwired: 9 in, 1 out]
      }
      event "Needle Alignment": Value Change {
        (unwired) "Needle Alignment in progress ...." ("String")
        # "CF height"
        # "surface z offset"
        # "first needle park position\nneedle gap on Z value : 0.5 mm"
        # "Syringe-camera offset"
        n247 = event-data() -> ()  [unwired: 1 in, 6 out]
        n248 = Array Subset(array=w743, index (row)=0, length (row)=1 ("length")) -> (w746:dbl[][])  [unwired: 2 in]
        n249 = Reshape Array(w746, 4 ("dimension size")) -> (w745:dbl[])
        n250 = Index Array(array=w745, index=2) -> (element=w742:dbl)
        n251 = call-poly <vilib>:"Read Delimited Spreadsheet.vi"("file path (dialog if empty)"=path "D:/INTT/V1/Assembly Data/Tool Offsets/Dispense Tip Offset.txt", "number of rows (all:-1)"=-1) -> ("first row"=w793:dbl[])  [unwired: 8 in, 5 out]
        n252 = Index Array(array=w793, index #1=0 ("index"), index #2=1 ("index")) -> (element #1=w788:dbl, element #2=w787:dbl)
        n253 = Add(x=14.2 ("element"), y=w751) -> (x+y=w753:dbl)
        n254 = Add(x=w742, y=w753) -> (x+y=w752:dbl)
        n255 = Build Array(436.638, 1040.76, w752, 0.0 ("element")) -> (w750:dbl[])
        n256 = Build Array(w788, w787, 0.0 ("element"), 0.0 ("element")) -> (w762:dbl[])
        n257 = call "XYZTheta Go.vi"("XYZTheta In"=w750, "Motion in"=w777) -> ("error out"=w786:errorcluster, "XYZTheta Out"=w767:dbl[], "Motion out"=w776:refnum<class "Motion.lvclass">)  [unwired: 7 in]
        n258 = call "Display Message to User10"("error in (no error)"=w786) -> ("error out"=w783:errorcluster)  [unwired: 9 in, 1 out]
        n259 = call-dynamic "Z Go.vi"("error in (no error)"=w783, "Speed"=20.0, "Position"=0.0, "Motion in"=w776) -> ("Motion out"=w775:refnum<class "Motion.lvclass">)  [unwired: 6 in, 1 out]
        n260 = Replace Array Subset(array=w767, new element=0.0 ("new element/subarray"), index=2) -> (w764:dbl[])
        n261 = call "Joystick and Camera - external Connection.vi"("Motion in"=w775, "XYZTheta"=w764, "Measurement Point"="Touch Needle on a surface") -> ("Motion out"=w773:refnum<class "Motion.lvclass">, "Gantry"=w763:dbl[])  [unwired: 4 in, 2 out]
        n262 = Subtract(x=w763, y=w762) -> (x-y=w761:dbl[])
        n263 = call "Joystick and Camera - external Connection.vi"("Motion in"=w773, "XYZTheta"=w761, "Measurement Point"="Measure the touch spot with camera") -> ("Motion out"=w769:refnum<class "Motion.lvclass">, "Gantry"=w772:dbl[])  [unwired: 4 in, 2 out]
        n264 = Subtract(x=w763, y=w772) -> (x-y=w771:dbl[])
        n265 = call-poly <vilib>:"Write Delimited Spreadsheet.vi"("file path (dialog if empty)"=path "D:/INTT/V1/Assembly Data/Tool Offsets/Dispense Tip Offset.txt", "1D data"=w771, "append to file? (new file:F)"=FALSE) -> ()  [unwired: 11 in, 2 out]
      }
      event "Pick and place": Value Change {
        (unwired) "PICK and PLACE samples ..." ("String")
        n266 = event-data() -> ()  [unwired: 1 in, 6 out]
        n267 = case shown="True" w799 {
          tunnel: w805 -> [w928 w950]
          tunnel: [w927 w949] -> w797
          frame False {
            n268 = Array Subset(array=w928, index (row)=0 ("index"), length (row)=1 ("length")) -> (w930:dbl[][])  [unwired: 2 in]
            n269 = Build Array(11.75 ("element"), 173.55 ("element"), 0.0 ("element"), 0.0 ("element")) -> (w934:dbl[])
            n270 = Reshape Array(w930, 4 ("dimension size")) -> (w929:dbl[])
            n271 = Add(x=w934, y=w929) -> (x+y=w927:dbl[])
          }
          frame True {
            n272 = Array Subset(array=w950, index (row)=0 ("index"), length (row)=1 ("length")) -> (w940:dbl[][])  [unwired: 2 in]
            n273 = Build Array(11.75 ("element"), 56.85 ("element"), 0.0 ("element"), 0.0 ("element")) -> (w944:dbl[])
            n274 = Reshape Array(w940, 4 ("dimension size")) -> (w939:dbl[])
            n275 = Add(x=w944, y=w939) -> (x+y=w949:dbl[])
          }
        }
        n276 = call-poly <vilib>:"Read Delimited Spreadsheet.vi"("file path (dialog if empty)"=path "D:/INTT/V1/Assembly Data/Tool Offsets/Bellows Tool Offset.txt", "number of rows (all:-1)"=-1) -> ("first row"=w820:dbl[])  [unwired: 8 in, 5 out]
        n277 = Index Array(array=w820, index #1=0 ("index"), index #2=1 ("index"), index #3=2 ("index")) -> (element #1=w816:dbl, element #2=w815:dbl, element #3=w814:dbl)
        n278 = for {
          N: 1 -> [_]
          tunnel: w823 -> [w832]
          tunnel: [w853] -> w813
          tunnel: w812 -> [w825] mode=indexing
          tunnel: [w841] -> w808
          tunnel: w809 -> [w831]
          tunnel: w816 -> [w855]
          tunnel: w815 -> [w854]
          tunnel: w814 -> [w852]
          tunnel: w801 -> [w847]
          tunnel: w807 -> [w834]
          tunnel: w797 -> [w833]
          tunnel: w803 -> [w829]
          tunnel: w798 -> [w824]
          w843 = 0 ("Write")
          w846 = TRUE ("Write Value")
          # "putback pickup tool"
          # "pickup tool"
          # "pickup tool height offset"
          # "Pick up PICKUP TOOL"
          # "Pick up CHIPs/Sensor and place on HDI"
          n279 = Build Array(w855, w854, w852, 0.0 ("element")) -> (w826:dbl[])
          n280 = Add(x=w825, y=w826) -> (x+y=w827:dbl[])
          n281 = call "XYZTheta-2Zspeed Go.vi"("XYZTheta In"=w827, "Motion in"=w832) -> ("error out"=w830:errorcluster, "Motion out"=w828:refnum<class "Motion.lvclass">)  [unwired: 7 in, 1 out]
          n282 = call "WriteReadWait.vi"("Read Value"=w846, "Write Value"=w846, "error in (no error)"=w830, "Read"=w843, "Write"=w843, "I-O in"=w831) -> ("error out"=w845:errorcluster, "I-O out"=w844:refnum<class "NI-DAQ.lvclass">)  [unwired: 4 in]
          n283 = Replace Array Subset(array=w826, new element=-16.0 ("t"), index=2) -> (w850:dbl[])
          n284 = for {
            N: w847 -> [_]
            tunnel: w828 -> [w874]
            tunnel: w850 -> [w873]
            tunnel: w845 -> [w872]
            tunnel: [w871] -> w856
            tunnel: w844 -> [w870]
            tunnel: [w869] -> w842
            tunnel: [w868] -> w849
            tunnel: w834 -> [w865]
            tunnel: w833 -> [w862]
            tunnel: w829 -> [w864] mode=indexing
            tunnel: w824 -> [w863] mode=indexing
            n285 = flat-sequence {
              tunnel: [w894] -> w875
              tunnel: w874 -> [w893]
              tunnel: w873 -> [w892]
              tunnel: w872 -> [w890]
              tunnel: w870 -> [w882]
              tunnel: [w889] -> w867
              tunnel: [w886] -> w866
              tunnel: w865 -> [w879]
              tunnel: w862 -> [w885]
              tunnel: w875 -> [w914]
              tunnel: [w926] -> w871
              tunnel: [w925] -> _
              tunnel: [w921] -> w869
              tunnel: [w918] -> w868
              tunnel: w867 -> [w923]
              tunnel: w866 -> [w919]
              tunnel: w864 -> [w920]
              tunnel: w863 -> [_]
              tunnel: w862 -> [w895]
              frame #0 {
                w880 = FALSE ("Write Value")
                w887 = TRUE ("Write Value")
                w888 = 1 ("Write")
                # "pickup module"
                # "release module"
                # "pickup sample from tray"
                n286 = Add(x=w885, y=w892) -> (x+y=w891:dbl[])
                n287 = call "XYZTheta-2Zspeed Go.vi"("error in (no error)"=w890, "XYZTheta In"=w891, "Motion in"=w893) -> ("error out"=w883:errorcluster, "Motion out"=w894:refnum<class "Motion.lvclass">)  [unwired: 6 in, 1 out]
                n288 = call "Time Delay"("error in (no error)"=w883) -> ("error out"=w876:errorcluster)  [unwired: 10 in]
                n289 = call "0"("error in (no error)"=w876) -> ("error out"=w877:errorcluster)  [unwired: 9 in, 1 out]
                n290 = call "WriteReadWait.vi"("Read Value"=w880, "Write Value"=w880, "error in (no error)"=w877, "Read"=w879, "Write"=w879, "I-O in"=w882) -> ("error out"=w878:errorcluster, "I-O out"=w881:refnum<class "NI-DAQ.lvclass">)  [unwired: 4 in]
                n291 = call "Time Delay3"("error in (no error)"=w878) -> ("error out"=w884:errorcluster)  [unwired: 10 in]
                n292 = call "WriteReadWait.vi"("Read Value"=w887, "Write Value"=w887, "error in (no error)"=w884, "Read"=w888, "Write"=w888, "I-O in"=w881) -> ("error out"=w886:errorcluster, "I-O out"=w889:refnum<class "NI-DAQ.lvclass">)  [unwired: 4 in]
              }
              frame #1 {
                w922 = 1 ("Write")
                w924 = FALSE ("Write Value")
                # "lift for chip/sensor thickness"
                # "place sample on HDI"
                n293 = Add(x=w920, y=dbl[] [0.0, 0.0, -16.0, 0.0]) -> (x+y=w912:dbl[])
                n294 = call-dynamic "Get Current Position.vi"("Motion in"=w914) -> ("XYZTheta Out"=w910:dbl[], "Motion out"=w913:refnum<class "Motion.lvclass">)  [unwired: 8 in, 1 out]
                "gantry position test" <- w910
                n295 = Array Subset(array=w895, index=0, length=2) -> (w899:dbl[])
                n296 = Build Array (concatenate)(w899, 0.0 ("element"), 0.0 ("element")) -> (w898:dbl[])
                n297 = Subtract(x=w912, y=w898) -> (x-y=w911:dbl[])
                "displacement" <- w911
                n298 = Array Subset(array=w910, index=0, length=2) -> (w905:dbl[])
                n299 = Build Array (concatenate)(w905, 0.0 ("element"), 0.0 ("element")) -> (w904:dbl[])
                n300 = Add(x=w904, y=w911) -> (x+y=w897:dbl[])
                "stave target position" <- w897
                n301 = call "XYZTheta-2Zspeed Go.vi"("error in (no error)"=w919, "XYZTheta In"=w897, "Motion in"=w913) -> ("error out"=w917:errorcluster, "XYZTheta Out"=w925:dbl[], "Motion out"=w926:refnum<class "Motion.lvclass">)  [unwired: 6 in]
                n302 = call "1"("error in (no error)"=w917) -> ("error out"=w916:errorcluster)  [unwired: 9 in, 1 out]
                n303 = call "Time Delay6"("error in (no error)"=w916) -> ("error out"=w915:errorcluster)  [unwired: 10 in]
                n304 = call "WriteReadWait.vi"("Read Value"=w924, "Write Value"=w924, "error in (no error)"=w915, "Read"=w922, "Write"=w922, "I-O in"=w923) -> ("error out"=w918:errorcluster, "I-O out"=w921:refnum<class "NI-DAQ.lvclass">)  [unwired: 4 in]
              }
            }
          }
          n305 = call "XYZTheta-2Zspeed Go.vi"("error in (no error)"=w849, "XYZTheta In"=w827, "Motion in"=w856) -> ("error out"=w837:errorcluster, "Motion out"=w860:refnum<class "Motion.lvclass">)  [unwired: 6 in, 1 out]
          n306 = call "Time Delay9"("error in (no error)"=w837) -> ("error out"=w839:errorcluster)  [unwired: 10 in]
          n307 = call-dynamic "Digital Write 1 Channel.vi"("DAQ Module"=0, "error constant"=w839, "Value"=FALSE, "Channel"=0, "NI-DAQ.lvclass"=w842) -> ("error IO"=w838:errorcluster, "NI-DAQ.lvclass 2"=w841:refnum<class "NI-DAQ.lvclass">)  [unwired: 5 in]
          n308 = call "Time Delay10"("error in (no error)"=w838) -> ("error out"=w857:errorcluster)  [unwired: 10 in]
          n309 = call-dynamic "Z Go.vi"("error in (no error)"=w857, "Speed"=10.0, "Position"=0.0 ("new element/subarray"), "Motion in"=w860) -> ("Motion out"=w853:refnum<class "Motion.lvclass">)  [unwired: 6 in, 1 out]
        }
      }
      event "GOTO": Value Change {
        (unwired) "GOING to a position" ("String")
        n310 = event-data() -> ()  [unwired: 1 in, 6 out]
        n311 = call "XYZTheta Go.vi"("XYZTheta In"="Parking position", "Motion in"=w957) -> ("Motion out"=w955:refnum<class "Motion.lvclass">)  [unwired: 7 in, 2 out]
      }
      event "READ Position": Value Change {
        n312 = event-data() -> ()  [unwired: 1 in, 6 out]
        n313 = call-dynamic "Get Current Position.vi"("Motion in"=w976) -> ("XYZTheta Out"=→"Gantry current position":dbl[], "Motion out"=w975:refnum<class "Motion.lvclass">)  [unwired: 8 in, 1 out]
      }
      event "HDI vacuum": Value Change {
        n314 = event-data() -> ()  [unwired: 1 in, 6 out]
        n315 = call "WriteReadWait.vi"("Read Value"="vacuum", "Write Value"="vacuum", "Read"=w988, "Write"=w988, "I-O in"=w991) -> ("error out"=w989:errorcluster, "I-O out"=w978:refnum<class "NI-DAQ.lvclass">)  [unwired: 5 in]
        n316 = call "Time Delay2"("error in (no error)"=w989) -> ()  [unwired: 10 in, 1 out]
      }
      event Timeout {
        n317 = event-data() -> ()  [unwired: 1 in, 3 out]
        n318 = call-dynamic "Digital Read 1 Channel.vi"("Read"=w1003, "NI-DAQ in"=w1004) -> ("Value"=→"Status":bool, "NI-DAQ out"=w1002:refnum<class "NI-DAQ.lvclass">)  [unwired: 7 in, 1 out]
      }
    }
    "Measured HDI size" <- w24
    "module positions on stave" <- w25
    "Stave mark" <- w23
    "measured HDI top-left position" <- w20
    n319 = feedback-in #1(w24) -> ()
    n320 = feedback-in #2(w23) -> ()
    n321 = feedback-in #3(w20) -> ()
    n322 = feedback-in #4(w9) -> ()
    n323 = feedback-in #5(w36) -> ()
    n324 = feedback-in #6(w33) -> ()
    n325 = feedback-in #7(w41) -> ()
    n326 = feedback-in #8(w25) -> ()
    n327 = feedback-in #9(w42) -> ()
    "# of tasks excuted" <- w38
  }
  n328 = call-dynamic "Disconnect.vi"("Controller in"=w4) -> ()  [unwired: 9 in, 1 out]
  n329 = call-dynamic "Disconnect.vi"("I-O in"=w1) -> ()  [unwired: 9 in, 1 out]
